vi "CSM - Running Log - DebugTool (CSMized).vi"() -> ()   [LabVIEW 2017]
doc: "Real-time tool for viewing the running log of the entire CSM program."
uses:
  Utility/_support/Periodic String Filter Level.ctl
  _Support/Typedef/_CSM_GlobalLog_MSG.ctl
  _Support/Typedef/_CSM_Response Source Message.ctl
  _Support/Typedef/_CSM_GlobalLog_MSG_TYPE.ctl
  _Support/GlobalEvent/GEvt-Generate with Rule Check.vi
  AdvanceAPI/CSM - Revert Arguments-Safe String.vi
  AdvanceAPI/CSM - Compact Multiple States.vi
  AdvanceAPI/CSM - Make String Arguments Safe.vi
  AdvanceAPI/CSM - Keywords.vi
  _Support/GlobalEvent/LogFilter/LogFilter - Check.vi
  _Support/GlobalEvent/FGV-GEvt Refs.vi
  _Shared/Trim Single-line Text.vi
  _Support/GlobalEvent/LogFilter/LogFilter.lvclass
  Communicable State Machine.lvlib
  addons/Logger/CSM File Logger.lvlib
  _Support/csm-tool-support.lvlib
  _csmHelper/API with lvcsm Support/CSM-Helper API with lvcsm Support.lvlib
panel:
  in  "Check Periodic Messages":bool
  in  "Filter Peroid Logs":bool
  in  "Record.Stop":bool
  in  "Record.Start":bool
  in  "BackTop":bool
  in  "Toolbar.History Length(char)":i32=50000 caption="History(char)" min=1000 max=100000000 step=1
  in  "Clear":bool
  in  "CSM":string(combo)
  in  "Search Button":bool
  in  "Toolbar.Open BD":bool
  in  "Toolbar.Open FP":bool
  in  "Periodic":bool
  in  "Check Peroid(s)":dbl=3.0
  in  "Threashold(#/s)":dbl=0.5
  in  "Periodic Info":bool=TRUE
  out "Handling Speed(#/s)":dbl
  in  "Level":T1
  out "LogInQ":i32
  out "State History":string
  in  "Tab":enum32{"Error History", "Broadcast Registry"}(tab)
  out "Error History":string
  out "Broadcast Registry":string[][](table)
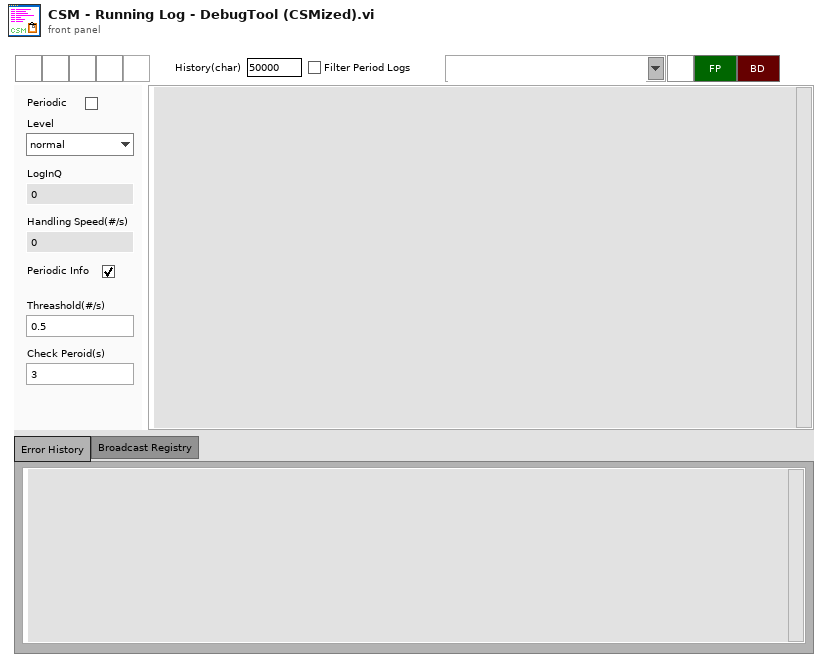
[diagram p1: front panel]
types:
  T1 = typedef "Communicable State Machine.lvlib/Periodic String Filter Level.ctl" = enum16{"normal", "L1", "L2", "L3", "L4"}
  T2 = enum32{"Invalid", "Standard", "Closed", "Hidden", "Minimized", "Maximized"}
  T3 = enum32{"invalid app kind", "Development System", "Run Time System", "Student Edition", "Embedded LabVIEW", "Evaluation", "Custom"}
  T4 = typedef "Communicable State Machine.lvlib/_CSM_Response Source Message.ctl" = cluster{"‘State":string, "’Arguments":string, "’Error":errorcluster}
  T5 = typedef "LVPoint32TypeDef.ctl" = cluster{"Horizontal":i32, "Vertical":i32}
  T6 = cluster{"Shift":bool, "Ctrl":bool, "Alt":bool, "Cmd":bool, "Opt":bool}
  T7 = cluster{"Core":cluster{"Current VI Reference":refnum<vi>, "Close Panel on Exit?":bool}, "Toolbar.Advance":refnum<vi>[], "LoggerWatchDogQueue":refnum<queue>, "LogFile":path}
  T8 = cluster{"Current VI Reference":refnum<vi>, "Close Panel on Exit?":bool}
  T9 = typedef "Communicable State Machine.lvlib/CSM - Broadcast Message Type.ctl" = enum16{"Status", "Interrupt(High)"}
  T10 = cluster{"Status":string, "Source CSM":string, "Target CSM":string, "Target API":string, "Priority":T9}[]
  T11 = cluster{"threashold(#/s)":dbl, "Check Peroid(s)":dbl}
  T12 = typedef "Communicable State Machine.lvlib/_CSM_GlobalLog_MSG.ctl" = cluster{"Name(\"\" to use uuid)":string, "Current State":string, "Arguments":string, "Source Message":T4, "Source Module":string, "Complete(T)/Start(F)":bool, "LogType":T13, "Time Stamp":timestamp}
  T13 = typedef "Communicable State Machine.lvlib/_CSM_GlobalLog_MSG_TYPE.ctl" = enum16{"User Log", "State Change", "Status", "Interrupt", "Register", "Unregister", "Error Log", "Module Created", "Module Destroyed"}
  T14 = cluster{"Threashold(#/s)":dbl, "Check Peroid(s)":dbl}
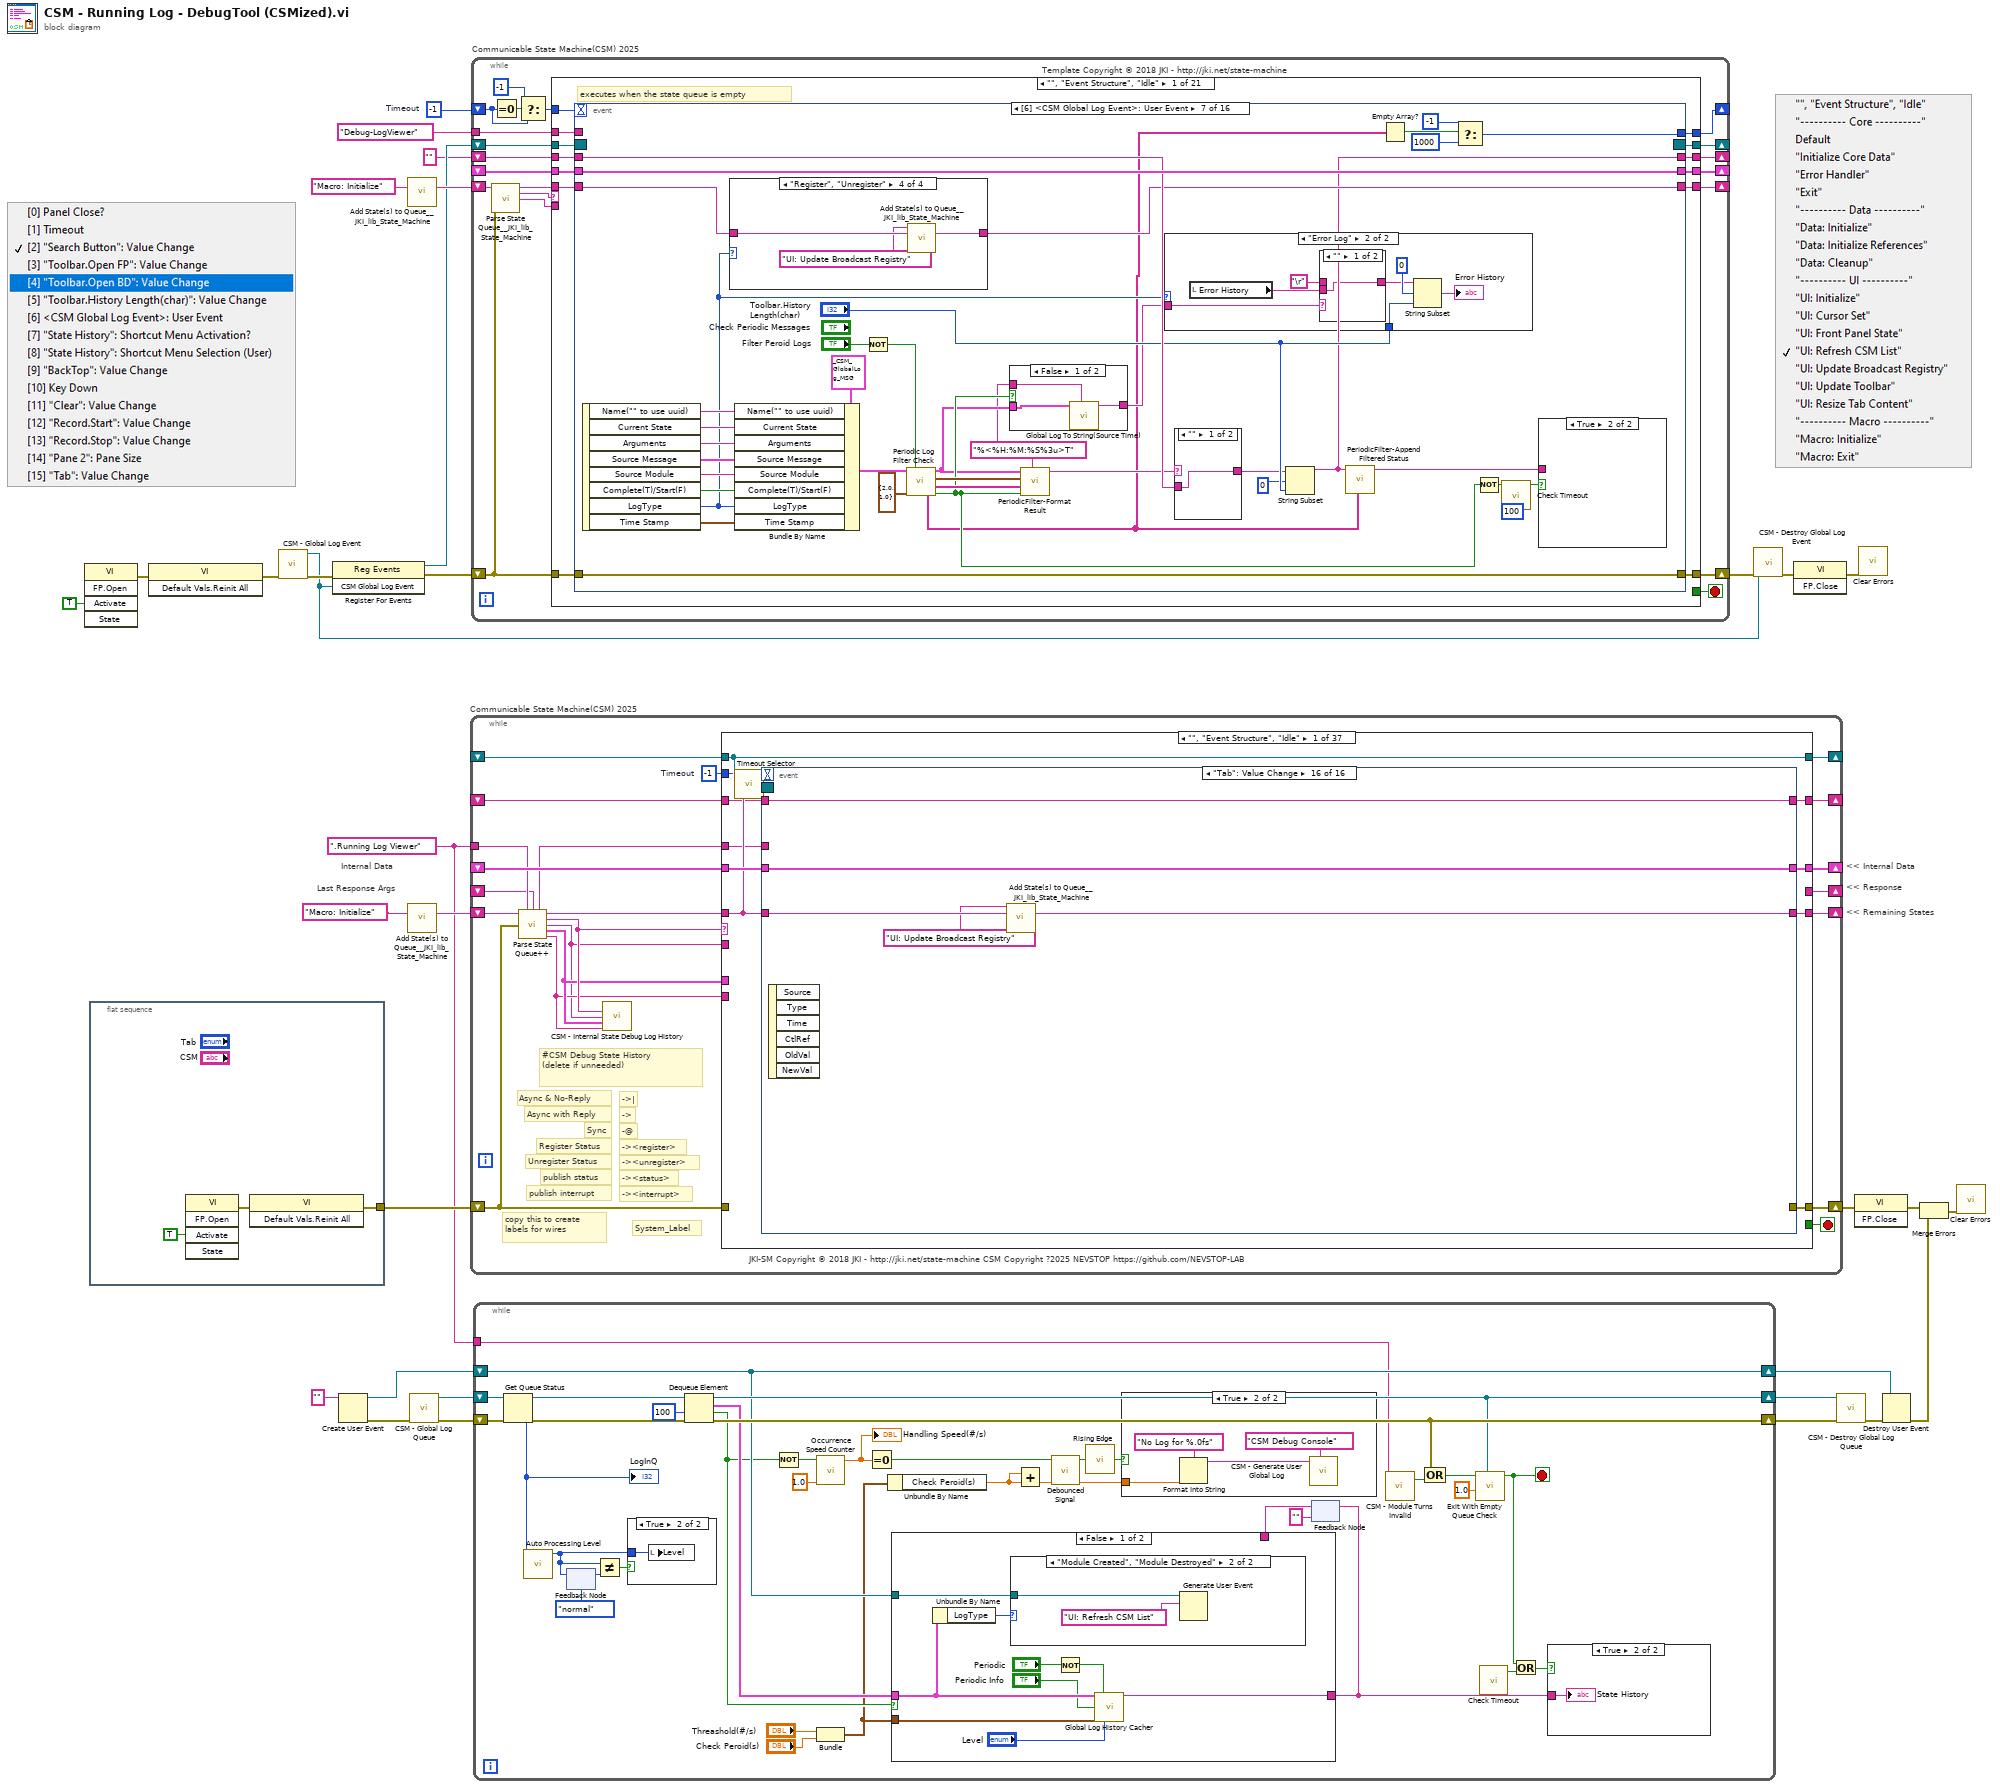
[diagram p0: block diagram]
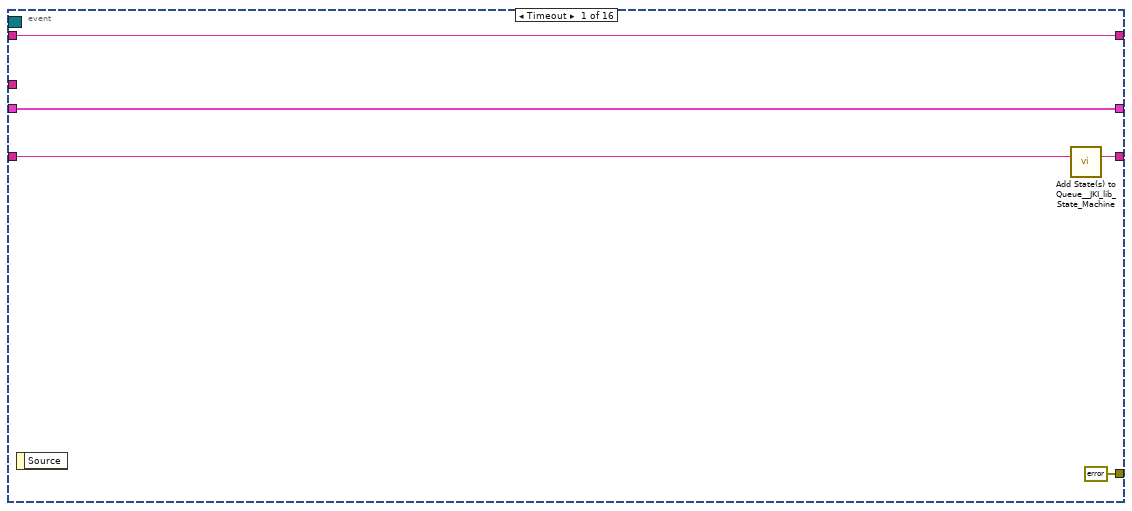
[diagram p7: hidden frame]
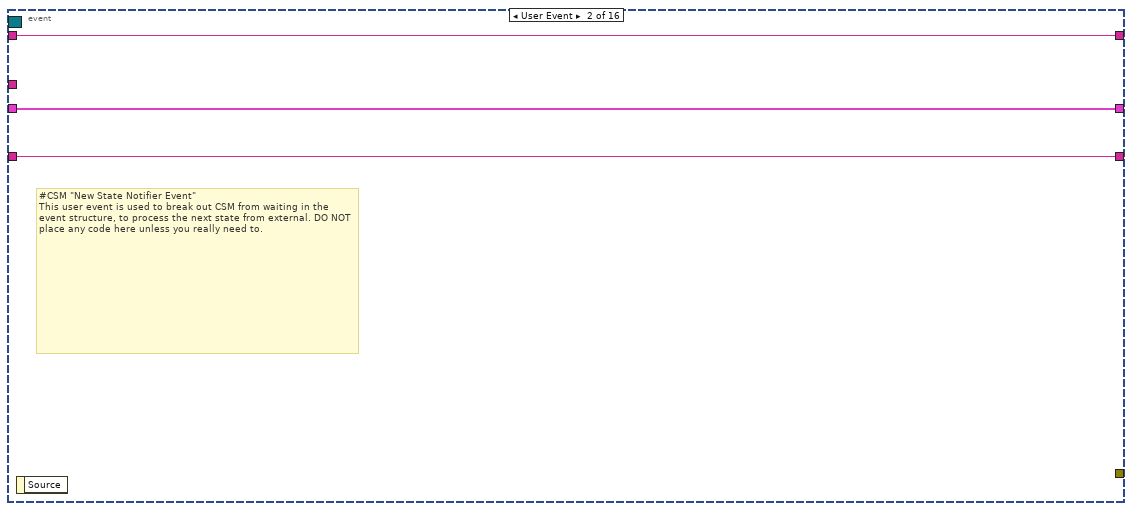
[diagram p8: hidden frame]
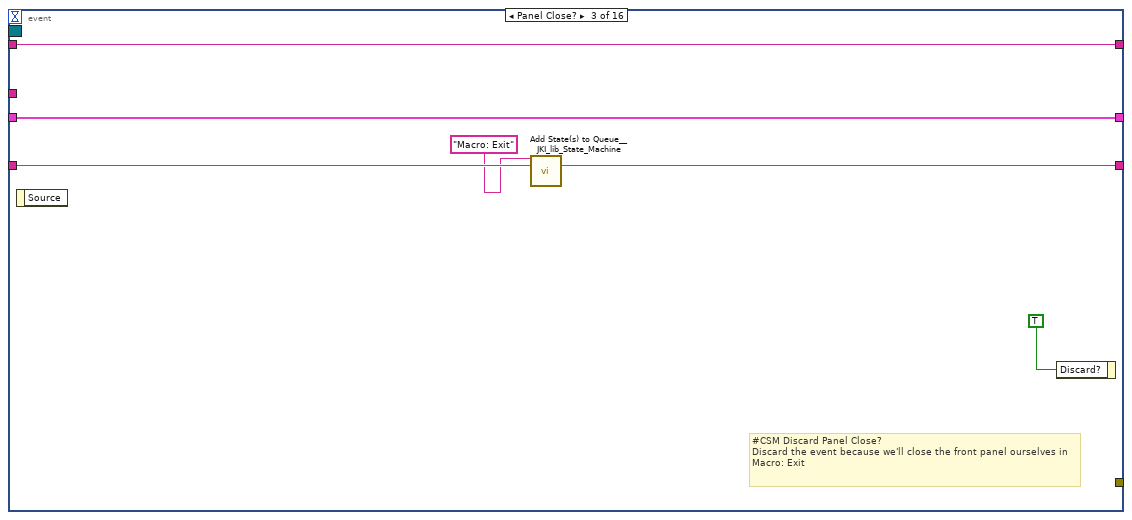
[diagram p9: hidden frame]
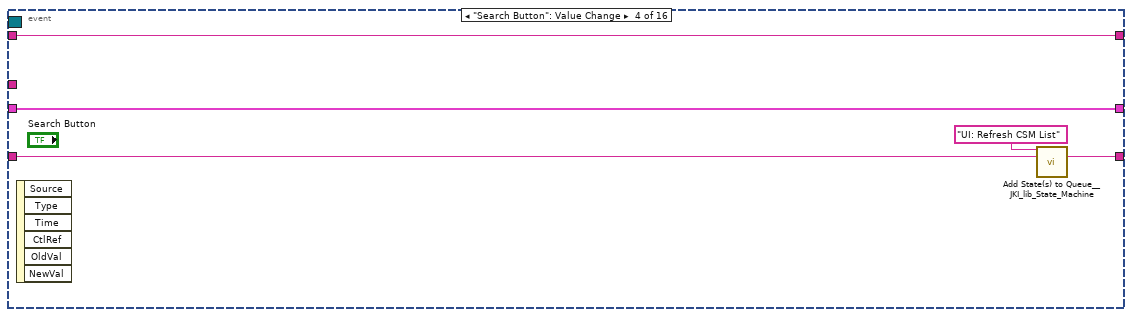
[diagram p10: hidden frame]
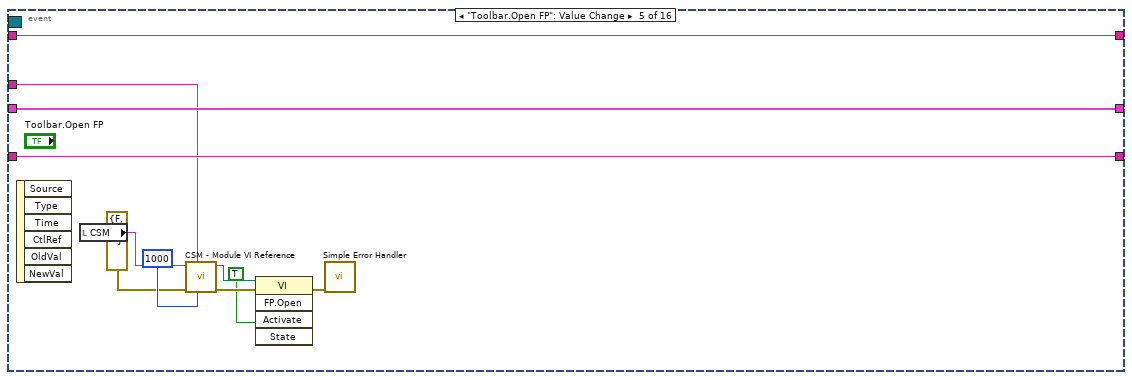
[diagram p11: hidden frame]
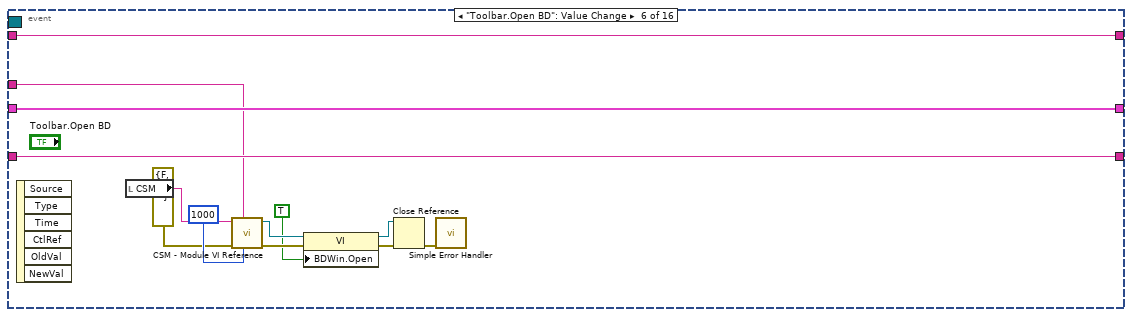
[diagram p12: hidden frame]
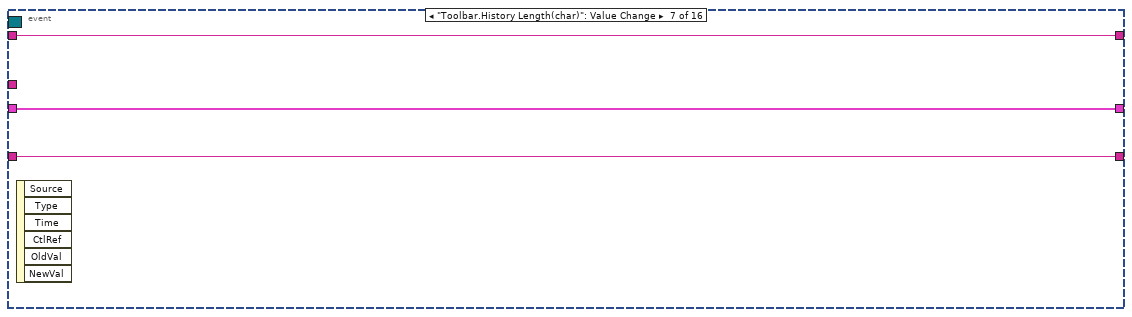
[diagram p13: hidden frame]
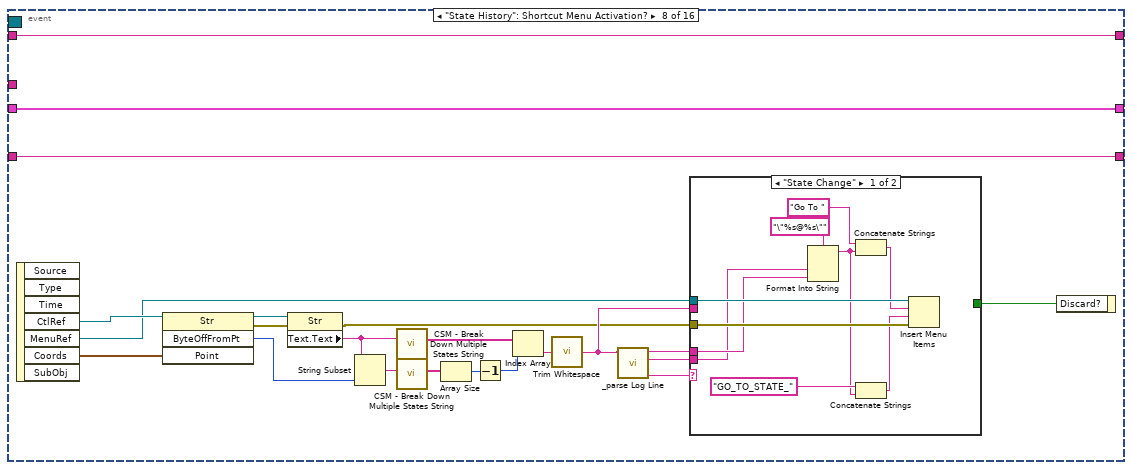
[diagram p14: hidden frame]
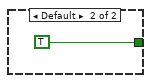
[diagram p15: hidden frame]
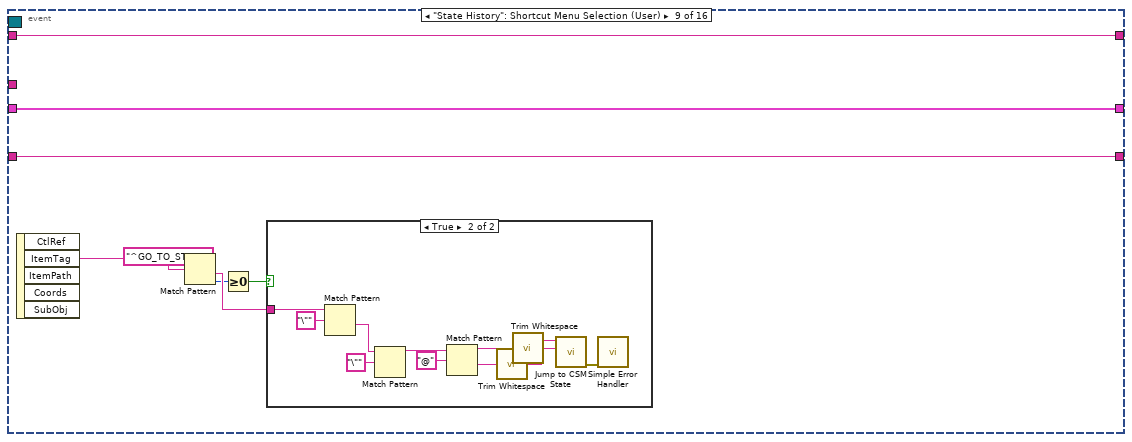
[diagram p16: hidden frame]
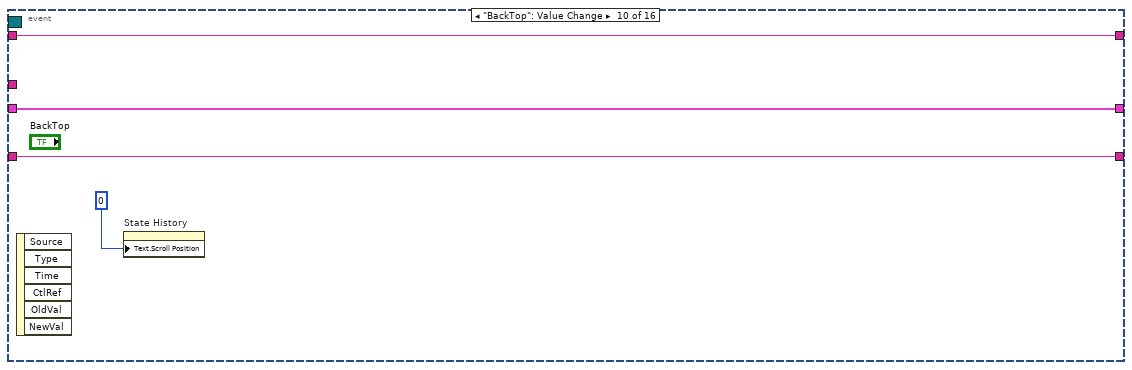
[diagram p18: hidden frame]
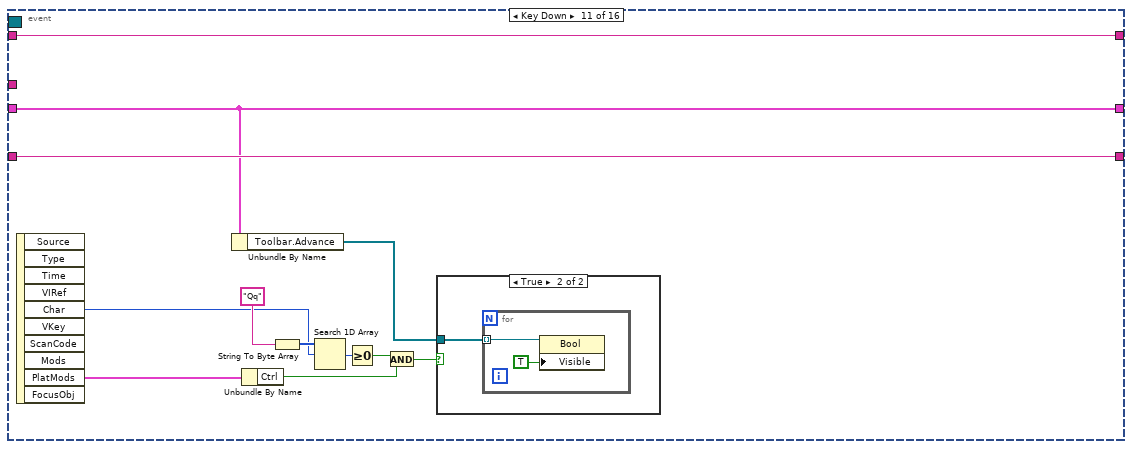
[diagram p19: hidden frame]
diagram:
  w7 = ".Running Log Viewer" ("Name(\"\" to use uuid)")
  w18 = -1  # Timeout
  # "Last Response Args"
  # "Internal Data"
  # "<< Internal Data"
  # "<< Response"
  # "<< Remaining States"
  n1 = invoke class="VI" method="FP.Open"("Activate"=TRUE ("Activate?")) -> (error out=w31:errorcluster)  [unwired: 4 in, 4 out]
  n2 = flat-sequence {
    tunnel: [w33] -> w15
    frame #0 {
      n3 = invoke class="VI" method="FP.Open"("Activate"=TRUE ("Activate?")) -> (error out=w35:errorcluster)  [unwired: 4 in, 4 out]
      n4 = invoke class="VI" method="Default Vals.Reinit All"(error in=w35) -> (error out=w33:errorcluster)  [unwired: 2 in, 2 out]
    }
  }
  n5 = invoke class="VI" method="Default Vals.Reinit All"(error in=w31) -> (error out=w25:errorcluster)  [unwired: 2 in, 2 out]
  n6 = call "CSM - Global Log Event.vi"("Error in"=w25) -> ("Error out"=w29:errorcluster, "CSM Global Log Event"=w28:refnum<user-event>)  [unwired: 9 in]
  n7 = register-events(error in=w29, w28) -> (reference out=w23:refnum<event-registration>, error out=w24:errorcluster)  [unwired: 1 in]
  n8 = Create User Event(user event datatype="" ("UserEvent")) -> (user event=w8:refnum<user-event>, error out=w9:errorcluster)  [unwired: 1 in]
  n9 = call <vilib>:"Add State(s) to Queue__JKI_lib_State_Machine.vi"("State(s) in (\"\")"="Macro: Initialize") -> ("States Out"=w27:string)  [unwired: 14 in]
  n10 = call <vilib>:"Add State(s) to Queue__JKI_lib_State_Machine.vi"("State(s) in (\"\")"="Macro: Initialize" ("Init State(\"Macro: Initialize\")")) -> ("States Out"=w17:string)  [unwired: 14 in]
  n11 = call "CSM - Global Log Queue.vi"("Error in"=w9) -> ("Error out"=w11:errorcluster, "GlobalEvent Queue"=w12:refnum<queue>)  [unwired: 9 in]
  n12 = while "Communicable State Machine(CSM) 2025" {
    shift-right: [w51] -> _
    shift-left: _ -> [w50]
    shift-right: [w54] -> w13
    shift-left: w15 -> [w48]
    shift-right: [w53] -> _
    shift-left: w17 -> [w55]
    tunnel: w7 -> [w44]
    shift-right: [w47] -> _
    shift-left: _ -> [w39]
    shift-right: [w46] -> _
    shift-left: _ -> [w45]
    shift-right: [w37] -> _
    shift-left: _ -> [w36]
    stop <- w52 stop-if-true
    w49 = -1  # Timeout
    # "#CSM Debug State History\n(delete if unneeded)"
    # "-><interrupt>"
    # "-><status>"
    # "-><unregister>"
    # "-><register>"
    # "-@"
    # "->"
    # "->|"
    # "publish interrupt"
    # "publish status"
    # "Unregister Status"
    # "Register Status"
    # "Sync"
    # "Async with Reply"
    # "Async & No-Reply"
    # "copy this to create labels for wires"
    # "System_Label"
    # "JKI-SM Copyright © 2018 JKI - http://jki.net/state-machine CSM Copyright ?2025 NEVSTOP https://github.com/NEVSTOP-LAB"
    n13 = call "Parse State Queue++.vi"("State Queue"=w55, "Name(\"\" to use uuid)"=w44, "Response Arguments"=w39, "Previous Error"=w48) -> ("Name Used"=w40:string, "Remaining States"=w56:string, "Current State"=w43:string, "Arguments"=w38:string, ">> Response Source Message >>"=w42:T4, ">> Source CSM >>"=w41:string)  [unwired: 6 in]
    n14 = call "CSM - Internal State Debug Log History.vi"("State"=w43, "Arguments (\"\")"=w38, ">> Response Source Message >>"=w42, "Source (\"\")"=w41) -> ()  [unwired: 11 in, 1 out]
    n15 = case shown="\"\", \"Event Structure\", \"Idle\"" w43 {
      selector: w43 -> [_ _ _ w237 _ _ _ _ _ _ _ _ _ _ _ _ _ _ _ _ _ _ _ _ _ _ _ _ _ _ _ _ _ _ _ _ _]
      tunnel: w56 -> [w60 w227 w233 w243 w250 w257 w284 w293 w301 w312 w322 w336 w342 w347 w356 w364 w372 w377 w385 w390 w395 w400 w407 w419 w490 w498 w525 w548 w554 w560 w572 w576 w581 w585 w590 w595 w600]
      tunnel: w38 -> [_ _ _ _ _ w255 w280 w288 w297 w306 _ _ _ _ _ _ _ _ _ _ _ _ w403 w414 _ _ _ _ _ _ _ _ _ _ _ _ _]
      tunnel: w50 -> [w66 w226 w230 w241 w249 w263 w285 w291 w299 w310 w321 w330 w340 w345 _ w360 w368 w375 w384 w389 w393 w398 w405 w416 w489 w497 w508 w547 w552 w558 w570 w575 w580 w584 w588 w593 w598]
      tunnel: [w65 _ w231 w235 w251 errorcluster {"status"=FALSE, "code"=0, "source"=""} ("error out") w277 w287 w295 w309 _ _ _ _ _ w365 w369 _ w379 w388 _ _ w404 w417 w491 w493 w526 w549 _ _ _ _ _ _ _ _ _] -> w54
      tunnel: w48 -> [_ _ w231 w236 w251 w261 w278 w289 w296 _ _ _ _ _ _ w365 _ _ _ _ _ _ _ _ w491 _ w526 w549 _ _ _ _ _ _ _ _ _]
      tunnel: [w67 w227 w232 w242 w250 w259 w283 w292 w300 w313 w322 w335 w341 w346 w355 w364 w371 w376 w385 w390 w394 w399 w406 w418 w490 w498 w525 w548 w553 w559 w571 w576 w581 w585 w589 w594 w599] -> w53
      tunnel: [_ _ _ _ _ _ TRUE _ _ _ _ _ TRUE _ _ _ _ _ _ _ _ _ _ _ _ _ _ _ _ _ _ _ _ _ _ _ _] -> w52
      tunnel: [w64 w226 w230 w241 w249 w263 w285 w291 w299 w311 w321 w334 w340 w345 w354 w358 w368 w375 w384 w389 w393 w398 w405 w416 w489 w497 w508 w547 w552 w558 w570 w575 w580 w584 w588 w593 w598] -> w51
      tunnel: w49 -> [w62 _ _ _ _ _ _ _ _ _ _ _ _ _ _ _ _ _ _ _ _ _ _ _ _ _ _ _ _ _ _ _ _ _ _ _ _]
      tunnel: w41 -> [_ _ _ _ _ w254 _ _ _ w307 _ _ _ _ _ _ _ _ _ _ _ _ _ _ _ _ _ _ _ _ _ _ _ _ _ _ _]
      tunnel: w42 -> [_ _ _ _ _ w253 _ _ _ w308 _ _ _ _ _ _ _ _ _ _ _ _ _ _ _ _ _ _ _ _ _ _ _ _ _ _ _]
      tunnel: [_ _ _ "" w245 _ _ _ _ _ _ _ _ _ _ _ _ _ _ _ _ _ _ _ _ _ _ _ _ _ _ _ "API1 Response" _ _ _ _] -> w47
      tunnel: [w63 w225 w229 w239 w248 w262 w281 w290 w298 w314 w320 w324 w338 w344 w352 w363 w367 w374 w383 w387 w392 w397 w402 w413 w488 w496 w524 w546 w551 w556 w563 w574 w579 w583 w587 w592 w597] -> w46
      tunnel: w45 -> [w63 w225 w229 w239 w248 w262 w281 w290 w298 w314 w320 w324 w338 w344 w352 w363 w367 w374 _ w387 w392 w397 w402 w413 w488 w496 w524 w546 w551 w556 w563 w574 w579 w583 w587 w592 w597]
      tunnel: w40 -> [w59 _ _ w238 _ _ w279 _ _ _ _ _ _ _ _ _ _ _ w382 _ _ _ _ _ _ _ _ _ _ _ _ _ _ _ _ _ _]
      tunnel: [w58 w224 w228 w234 w244 w252 w276 w286 w294 w302 w319 w323 w337 w343 w348 w357 w366 w373 w378 w386 w391 w396 w401 w412 w480 w492 w507 w533 w550 w555 w561 w573 w577 w582 w586 w591 w596] -> w37
      tunnel: w36 -> [w57 w224 w228 w234 w244 w252 w276 w286 w294 w302 w319 w323 w337 w343 w348 w357 w366 w373 w378 w386 w391 w396 w401 w412 w480 w492 w507 w533 w550 w555 w561 w573 w577 w582 w586 w591 w596]
      frame "", "Event Structure", "Idle" {
        n16 = call "Timeout Selector.vi"("Remaining States"=w60, "Timeout Expected"=w62) -> ("Timeout"=w61:i32)  [unwired: 5 in]
        n17 = event shown="[15] \"Tab\": Value Change" {
          selector: w63 -> [_ _ _ _ _ _ _ _ _ _ _ _ _ _ _ _]
          dyn-events: _ -> [_ _ _ _ _ _ _ _ _ _ _ _ _ _ _ _]
          timeout: w61 -> [_ _ _ _ _ _ _ _ _ _ _ _ _ _ _ _]
          tunnel: w60 -> [w72 w74 w81 w85 w97 w110 w113 w135 w154 w169 w181 w187 w191 w206 w214 w220]
          tunnel: [w71 w74 w80 w84 w97 w110 w113 w135 w154 w169 w181 w187 w190 w205 w215 w221] -> w67
          tunnel: w66 -> [w70 w75 w79 w86 w96 w109 w112 w134 w153 w168 w171 w186 w193 w208 w218 w223]
          tunnel: [errorcluster {"status"=FALSE, "code"=0, "source"=""} ("error out") _ _ _ _ _ _ _ _ _ _ _ w188 _ _ _] -> w65
          tunnel: [w70 w75 w79 w86 w96 w109 w112 w134 w153 w168 w171 w186 w192 w207 w218 w223] -> w64
          tunnel: w59 -> [_ _ _ _ w88 w99 _ _ _ _ _ _ _ _ _ _]
          tunnel: [w68 w73 w76 w82 w87 w98 w111 w114 w147 w166 w170 w185 w203 w213 w217 w222] -> w58
          tunnel: w57 -> [w68 w73 w76 w82 w87 w98 w111 w114 w147 w166 w170 _ w203 w213 w217 w222]
          event Timeout {
            n18 = event-data() -> ()  [unwired: 1 in, 1 out]
            n19 = call <vilib>:"Add State(s) to Queue__JKI_lib_State_Machine.vi"("State(s) in (\"\")"=w72) -> ("States Out"=w71:string)  [unwired: 14 in]
          }
          event User Event {
            # "#CSM \"New State Notifier Event\"\nThis user event is used to break out CSM from waiting in the event structure, to process the next state from external. DO NOT place any code here unless you really need to."
            n20 = event-data() -> ()  [unwired: 1 in, 1 out]
          }
          event Panel Close? {
            # "#CSM Discard Panel Close?\nDiscard the event because we'll close the front panel ourselves in Macro: Exit"
            n21 = event-data() -> ()  [unwired: 1 in, 1 out]
            n22 = call <vilib>:"Add State(s) to Queue__JKI_lib_State_Machine.vi"("State(s) in Front (\"\")"="Macro: Exit", "State(s) in (\"\")"=w81) -> ("States Out"=w80:string)  [unwired: 13 in]
            n23 = event-data("Discard?"=TRUE) -> ()  [unwired: 1 in, 1 out]
          }
          event "Search Button": Value Change {
            n24 = event-data() -> ()  [unwired: 1 in, 6 out]
            n25 = call <vilib>:"Add State(s) to Queue__JKI_lib_State_Machine.vi"("State(s) in Front (\"\")"="UI: Refresh CSM List" ("State(s) in Front (\"\")"), "State(s) in (\"\")"=w85) -> ("States Out"=w84:string)  [unwired: 13 in]
          }
          event "Toolbar.Open FP": Value Change {
            n26 = event-data() -> ()  [unwired: 1 in, 6 out]
            n27 = local read "CSM"() -> (w93:string)
            n28 = call "CSM - Module VI Reference.vi"("Response Timeout(-2 using Global Settings)"=1000 ("Response Timeout(5000ms)"), "Current Module(\"\" to generate a ID)"=w88, "error in (no error)"=errorcluster {"status"=FALSE, "code"=0, "source"=""}, "CSM Name"=w93) -> ("error out"=w95:errorcluster, "CSM Module VIRef"=w94:refnum<vi>)  [unwired: 6 in]
            n29 = invoke on="Invoke Node" class="VI" method="FP.Open"(reference=w94, error in=w95, "Activate"=TRUE ("Activate?")) -> (error out=w92:errorcluster)  [unwired: 2 in, 4 out]
            n30 = call <vilib>:"Simple Error Handler.vi"("error in (no error)"=w92) -> ()  [unwired: 4 in, 5 out]
          }
          event "Toolbar.Open BD": Value Change {
            n31 = event-data() -> ()  [unwired: 1 in, 6 out]
            n32 = local read "CSM"() -> (w104:string)
            n33 = call "CSM - Module VI Reference.vi"("Response Timeout(-2 using Global Settings)"=1000 ("Response Timeout(5000ms)"), "Current Module(\"\" to generate a ID)"=w99, "error in (no error)"=errorcluster {"status"=FALSE, "code"=0, "source"=""}, "CSM Name"=w104) -> ("error out"=w108:errorcluster, "CSM Module VIRef"=w105:refnum<vi>)  [unwired: 6 in]
            n34 = property class="VI"(reference=w105, error in=w108, "BDWin.Open"=TRUE ("Block Diagram Window:Open")) -> (reference out=w106:refnum<vi>, error out=w107:errorcluster)
            n35 = Close Reference(reference=w106, error in (no error)=w107) -> (error out=w103:errorcluster)
            n36 = call <vilib>:"Simple Error Handler.vi"("error in (no error)"=w103) -> ()  [unwired: 4 in, 5 out]
          }
          event "Toolbar.History Length(char)": Value Change {
            n37 = event-data() -> ()  [unwired: 1 in, 6 out]
          }
          event "State History": Shortcut Menu Activation? {
            n38 = event-data() -> ("CtlRef"=w118:refnum<vi>, "MenuRef"=w116:refnum<k9>, "Coords"=w117:T5)  [unwired: 1 in, 4 out]
            n39 = invoke class="Str" method="ByteOffFromPt"(reference=w118, "Point"=w117) -> (reference out=w119:refnum<vi>, error out=w121:errorcluster, "ByteOffFromPt"=w120:i32)  [unwired: 2 in, 1 out]
            n40 = property class="Str"(reference=w119, error in=w121) -> (error out=w129:errorcluster, "Text.Text"=w123:string)  [unwired: 1 out]
            n41 = String Subset(string=w123, length (rest)=w120) -> (substring=w122:string)  [unwired: 1 in]
            n42 = call "CSM - Break Down Multiple States String.vi"("States"=w123) -> ("Multiple States"=w124:string[])  [unwired: 10 in]
            n43 = call "CSM - Break Down Multiple States String.vi"("States"=w122) -> ("Multiple States"=w125:string[])  [unwired: 10 in]
            n44 = Array Size(array=w125) -> (size(s)=w126:i32)
            n45 = Decrement(x=w126) -> (x-1=w127:i32)
            n46 = Index Array(array=w124, index=w127) -> (element=w128:string)
            n47 = call <vilib>:"Trim Whitespace.vi"("string"=w128) -> ("trimmed string"=w130:string)  [unwired: 1 in]
            n48 = call "_parse Log Line.vi"("string"=w130) -> ("LogType"=w131:string, "State"=w133:string, "CSM"=w132:string)  [unwired: 8 in]
            n49 = case shown="\"State Change\"" w131 {
              tunnel: w116 -> [w145 _]
              tunnel: w130 -> [_ _]
              tunnel: w129 -> [w143 _]
              tunnel: [_ TRUE] -> w115
              tunnel: w132 -> [w141 _]
              tunnel: w133 -> [w140 _]
              frame "State Change" {
                n50 = Format Into String(format string="\"%s@%s\"", w140, w141) -> (resulting string=w136:string)  [unwired: 2 in, 1 out]
                n51 = Concatenate Strings("Go To " ("format string"), w136) -> (w139:string)
                n52 = Concatenate Strings("GO_TO_STATE_" ("item tags"), w136) -> (w137:string)
                n53 = Insert Menu Items(6:w143, 7:w137, 8:w139, 9:w145) -> ()  [unwired: 2 in, 3 out]
              }
              frame Default {
              }
            }
            n54 = event-data("Discard?"=w115) -> ()  [unwired: 1 in, 1 out]
          }
          event "State History": Shortcut Menu Selection (User) {
            n55 = event-data() -> ("ItemTag"=w148:string)  [unwired: 1 in, 4 out]
            n56 = Match Pattern(string=w148, regular expression="^GO_TO_STATE") -> (after substring=w152:string, offset past match=w150:i32)  [unwired: 1 in, 2 out]
            n57 = Greater Or Equal To 0?(x=w150) -> (x >= 0?=w151:bool)
            n58 = case shown="True" w151 {
              tunnel: w152 -> [_ w165]
              frame False {
              }
              frame True {
                n59 = Match Pattern(string=w165, regular expression="\"") -> (after substring=w162:string)  [unwired: 1 in, 3 out]
                n60 = Match Pattern(string=w162, regular expression="\"") -> (before substring=w161:string)  [unwired: 1 in, 3 out]
                n61 = Match Pattern(string=w161, regular expression="@") -> (before substring=w159:string, after substring=w158:string)  [unwired: 1 in, 2 out]
                n62 = call <vilib>:"Trim Whitespace.vi"("string"=w158) -> ("trimmed string"=w156:string)  [unwired: 1 in]
                n63 = call <vilib>:"Trim Whitespace.vi"("string"=w159) -> ("trimmed string"=w157:string)  [unwired: 1 in]
                n64 = call "Jump to CSM State.vi"("State"=w157, "Name"=w156) -> ("Error out"=w155:errorcluster)  [unwired: 9 in]
                n65 = call <vilib>:"Simple Error Handler.vi"("error in (no error)"=w155) -> ()  [unwired: 4 in, 5 out]
              }
            }
          }
          event "BackTop": Value Change {
            n66 = event-data() -> ()  [unwired: 1 in, 6 out]
            n67 = property on="State History" class="Str"("Text.Scroll Position"=u32 0) -> ()  [unwired: 2 in, 2 out]
          }
          event Key Down {
            n68 = event-data() -> ("Char"=w173:i16, "PlatMods"=w172:T6)  [unwired: 1 in, 8 out]
            n69 = Unbundle By Name(w171) -> ("Toolbar.Advance"=w180:refnum<vi>[])
            n70 = Unbundle By Name(w172) -> ("Ctrl"=w178:bool)
            n71 = String To Byte Array(string="Qq") -> (unsigned byte array=w176:u8[])
            n72 = Search 1D Array(1D array=w176, element=w173) -> (index of element=w175:i32)  [unwired: 1 in]
            n73 = Greater Or Equal To 0?(x=w175) -> (x >= 0?=w174:bool)
            n74 = And(x=w174, y=w178) -> (x .and. y?=w179:bool)
            n75 = case shown="True" w179 {
              tunnel: w180 -> [_ w182]
              frame False {
              }
              frame True {
                n76 = for {
                  tunnel: w182 -> [w184] mode=indexing
                  n77 = property class="Bool"(reference=w184, "Visible"=TRUE) -> ()  [unwired: 1 in, 2 out]
                }
              }
            }
          }
          event "Clear": Value Change {
            w185 = "" ("String Cache")
            n78 = event-data() -> ()  [unwired: 1 in, 6 out]
            n79 = local write "State History"(w185) -> ()
            n80 = local write "Error History"(w185) -> ()
          }
          event "Record.Start": Value Change {
            n81 = event-data() -> ()  [unwired: 1 in, 6 out]
            n82 = Unbundle By Name(w193) -> ("Core.Current VI Reference"=w196:refnum<vi>)
            n83 = property class="VI"(reference=w196) -> (error out=w197:errorcluster, "OwningApp"=w198:refnum<vi>)  [unwired: 1 in, 1 out]
            n84 = property class="App"(reference=w198, error in=w197) -> (error out=w200:errorcluster, "Project.ActiveProject"=w199:refnum<vi>)  [unwired: 1 out]
            n85 = property class="Project"(reference=w199, error in=w200) -> ("Name"=w201:string)  [unwired: 2 out]
            n86 = String To Path(string=w201) -> (path=w202:path)
            n87 = call "CSM - Start File Logger.vi"("Log File Path"=w202) -> ("Error out"=w188:errorcluster, "LogFile"=w195:path, "WatchDogQueue"=w194:refnum<queue>)  [unwired: 8 in]
            n88 = Bundle By Name(cluster=w193, "LoggerWatchDogQueue"=w194, "LogFile"=w195) -> (w192:T7)
            n89 = call <vilib>:"Add State(s) to Queue__JKI_lib_State_Machine.vi"("State(s) in Front (\"\")"="UI: Update Toolbar" ("State(s) in Front (\"\")"), "State(s) in (\"\")"=w191) -> ("States Out"=w190:string)  [unwired: 13 in]
          }
          event "Record.Stop": Value Change {
            n90 = event-data() -> ()  [unwired: 1 in, 6 out]
            n91 = Unbundle By Name(w208) -> ("LoggerWatchDogQueue"=w212:refnum<queue>)
            n92 = Release Queue(queue=w212, force destroy? (F)=TRUE) -> (error out=w210:errorcluster)  [unwired: 1 in, 2 out]
            n93 = call <vilib>:"Clear Errors.vi"("error in (no error)"=w210) -> ()  [unwired: 5 in, 2 out]
            n94 = Bundle By Name(cluster=w208, "LogFile"=path "") -> (w207:T7)
            n95 = call <vilib>:"Add State(s) to Queue__JKI_lib_State_Machine.vi"("State(s) in Front (\"\")"="UI: Update Toolbar" ("State(s) in Front (\"\")"), "State(s) in (\"\")"=w206) -> ("States Out"=w205:string)  [unwired: 13 in]
          }
          event Pane Size {
            n96 = event-data() -> ()  [unwired: 1 in, 6 out]
            n97 = call <vilib>:"Add State(s) to Queue__JKI_lib_State_Machine.vi"("State(s) in (\"\")"=w214, "State(s) at Back (\"\")"="UI: Resize Tab Content" ("State(s) in Front (\"\")")) -> ("States Out"=w215:string)  [unwired: 13 in]
          }
          event "Tab": Value Change {
            n98 = event-data() -> ()  [unwired: 1 in, 6 out]
            n99 = call <vilib>:"Add State(s) to Queue__JKI_lib_State_Machine.vi"("State(s) in Front (\"\")"="UI: Update Broadcast Registry" ("State(s) in Front (\"\")"), "State(s) in (\"\")"=w220) -> ("States Out"=w221:string)  [unwired: 13 in]
          }
        }
      }
      frame "CSM Documentation" {
        # "#CSM State Syntax\n\n// Comment line, all text to the right of “//” will be ignored\n// Local Message Example\nDoSth: DoA >> Arguments\n\n// Sync Call Example\nAPI: xxxx >> Arguments -@ TargetModule\n\n// Async Call Example\nAPI: xxxx >> Arguments -> TargetModule\n\n// Async Call without Reply Example\nAPI: xxxx >> Arguments ->| TargetModule\n\n// Broadcast normal status:\nStatus >> StatusArguments  -><status>\n\n// Broadcast Interrupt status:\nInterrupt >> StatusArguments  -><interrupt>\n\n// Register Source Module's status to Handler Module\nStatus@Source Module >> Handler Module@Handler Module -><register>\n\n// Unegister Source Module's status\nStatus@Source Module >> Handler Module -><unregister>"
        # "#CSM README FIRST\n\nCommunicable State Machine(CSM) is a LabVIEW application framework that builds upon JKI State Machine(JKISM). It follows the pattern of JKISM and extends the keywords to describe message communication between modules, including concepts such as Sync-Message, Async-Message, Subscription/Unsubscription of status - essential elements for creating reusable code modules. For more information, please visit the CSM wiki: https://nevstop-lab.github.io/CSM-Wiki/\n\nFor instructions on JKI State Machine, visit: \n    http://jki.net/state-machine/\nFor information about CSM, visit: \n    https://github.com/NEVSTOP-LAB"
        # "#CSM \"Documentation\"\nCase for holding CSM Documenation"
      }
      frame "---------- Core ----------" {
        # "#CSM \"Category Seperator\"\nDo not put any code in this frame."
        n100 = call <vilib>:"Add State(s) to Queue__JKI_lib_State_Machine.vi"("State(s) in (\"\")"=w233) -> ("States Out"=w232:string)  [unwired: 14 in]
      }
      frame Default {
        # "#CSM \"Default\"\nthis is used to capture unhandled states and typos"
        n101 = call "CSM Unhandled State Error.vi"("error in (no error)"=w236, "Current State"=w237, "CSM Name"=w238) -> ("error out"=w235:errorcluster)  [unwired: 8 in]
        n102 = call <vilib>:"Add State(s) to Queue__JKI_lib_State_Machine.vi"("State(s) in (\"\")"=w243) -> ("States Out"=w242:string)  [unwired: 14 in]
      }
      frame "VI Reference" {
        n103 = Unbundle By Name(w249) -> ("Core"=w247:T8)
        n104 = Unbundle By Name(w247) -> ("Current VI Reference"=w246:refnum<vi>)
        n105 = call "CSM - Convert Data to HexStr.vi"("Variant"=w246) -> ("HEX String (0-9,A-F)"=w245:string)  [unwired: 8 in]
      }
      frame "Error Handler" {
        # "#CSM Disable this error dialog if you need"
        # "#CSM \"Error Handler\"\nYou can also output any states to clean-up after errors occur"
        # "Clear error"
        n106 = case shown="Error" w261 {
          selector: w261 -> [_ w270]
          tunnel: [w268 w272] -> w258
          tunnel: w257 -> [w268 w271]
          tunnel: [w267 w270] -> w256
          tunnel: w255 -> [w269 _]
          tunnel: w254 -> [_ _]
          tunnel: w253 -> [_ _]
          frame No Error {
            n107 = call "CSM - Convert Argument to Error.vi"("Argument"=w269) -> ("error"=w267:errorcluster)  [unwired: 4 in]
            n108 = flat-sequence {
              frame #0 {
                # "#CSM External Error Handler Case\nUsually, it's because This CSM register others' \"Error Occurred\" status with \"Error Handler\". If other CSM have any error, the error will be passed here for central handling."
              }
            }
          }
          frame Error {
            # "#CSM Internal Error Handler Case \nIf any error Occurred, \"Error Occurred\" \nstatus update will be broadcasted to system.\nParameter is Error Cluster."
            n109 = call "CSM - Convert Error to Argument.vi"("error"=w270) -> ("Argument"=w274:string)  [unwired: 4 in]
            n110 = call <vilib>:"Build State String with Arguments__JKI_lib_State_Machine.vi"("Arguments (\"\")"=w274, "State"="Error Occurred" ("Status with Arguments")) -> ("State with Arguments"=w273:string)  [unwired: 4 in]
            n111 = call "CSM - Broadcast Status Change.vi"("Status with Arguments"=w273, "State Queue"=w271) -> ("Remaining States"=w272:string)  [unwired: 13 in]
          }
        }
        n112 = disable-structure shown="Enabled" {
          disable-tunnel: w256 -> [w265 w266]
          frame Enabled {
            # "Unhandled Error -- Display it"
            n113 = call <vilib>:"General Error Handler.vi"("error in (no error)"=w265) -> ()  [unwired: 10 in, 5 out]
          }
          frame Disabled {
            n114 = call <vilib>:"Clear Errors.vi"("error in (no error)"=w266) -> ()  [unwired: 5 in, 2 out]
          }
        }
        n115 = call <vilib>:"Add State(s) to Queue__JKI_lib_State_Machine.vi"("State(s) in Front (\"\")"="// Post Error States", "State(s) in (\"\")"=w258) -> ("States Out"=w259:string)  [unwired: 13 in]
      }
      frame "Critical Error" {
        # "#CSM \"Critical Error\"\nWhen any un-recoverable error occurs, CSM goes into this case."
        # "#CSM Stop in Critical Error\nWhen Critical Error occurs, Stop the loop immediately. Do NOT change this unless you fully understand the impact."
        n116 = call "CSM Critical Error.vi"("error in (no error)"=w278, "Arugments(as Reason)"=w280, "CSM Name"=w279) -> ("error out"=w277:errorcluster)  [unwired: 8 in]
        n117 = call <vilib>:"Add State(s) to Queue__JKI_lib_State_Machine.vi"("State(s) in (\"\")"=w284) -> ("States Out"=w283:string)  [unwired: 14 in]
      }
      frame "Target Timeout Error" {
        # "#CSM \"Target Timeout Error\"\nWhen This CSM could not get the sync-call response in time, This CSM goes into this case."
        n118 = call "CSM Target Timeout Error.vi"("error in (no error)"=w289, "Arguments(as CSM Name)"=w288) -> ("error out"=w287:errorcluster)  [unwired: 9 in]
        n119 = call <vilib>:"Add State(s) to Queue__JKI_lib_State_Machine.vi"("State(s) in (\"\")"=w293) -> ("States Out"=w292:string)  [unwired: 14 in]
      }
      frame "Target Error" {
        # "#CSM \"Target Error\"\nWhen This CSM try to communicate with an un-existed CSM, This CSM goes into this case."
        n120 = call "CSM Target Error.vi"("error in (no error)"=w296, "Arguments(as CSM Name)"=w297) -> ("error out"=w295:errorcluster)  [unwired: 9 in]
        n121 = call <vilib>:"Add State(s) to Queue__JKI_lib_State_Machine.vi"("State(s) in (\"\")"=w301) -> ("States Out"=w300:string)  [unwired: 14 in]
      }
      frame "Async Response", "Response" {
        # "#CSM \"Async Response\"\nHandle Async-call Response (\"Async Response\" for ->)"
        # "#CSM \"Response\"\nHandle Sync-call Response (\"Response\" for -@)"
        n122 = Unbundle(w308) -> ("‘State"=w305:string, "’Arguments"=w304:string, "’Error"=w303:errorcluster)
        n123 = case shown="Default" w305 {
          tunnel: [w315] -> w313
          tunnel: w312 -> [w316]
          tunnel: [w318] -> w311
          tunnel: w310 -> [w318]
          tunnel: [w317] -> w309
          tunnel: w303 -> [w317]
          tunnel: w307 -> [_]
          tunnel: w306 -> [_]
          tunnel: w304 -> [_]
          frame Default {
            # "#CSM Response Comments\nAfter Message is executed, CSM goes to this state for receive the response.\n    For Async Message(->), \"Async Response\" is used. This CSM will goes to \"Async Message Posted\" immediately and receive the \"Async Response\" after the callee finishes the message.\n    For Sync Message(@),  This CSM will wait until the message is done and immediately goes to \"Response\""
            n124 = call <vilib>:"Add State(s) to Queue__JKI_lib_State_Machine.vi"("State(s) in (\"\")"=w316) -> ("States Out"=w315:string)  [unwired: 14 in]
          }
        }
      }
      frame "Async Message Posted" {
        # "#CSM \"Async Message Posted\"\nAfter Async Message is posted (-> or ->| ), CSM goes to this state for post-action.\nYou can use Argument - State to tell which Async Message is called."
      }
      frame "Initialize Core Data" {
        # "#CSM \"Initialize Core Data\"\nThis is used to determine panel behavior on exit"
        # "originally closed?"
        # "exe?"
        # "If panel starts closed or is an EXE, then close it when we exit"
        n125 = property class="VI"() -> ("FP.State"=w327:T2)  [unwired: 2 in, 2 out]
        n126 = property class="App"() -> ("App.Kind"=w333:T3)  [unwired: 2 in, 2 out]
        n127 = control-ref of="Current VI Reference"() -> (w328:refnum<vi>)
        n128 = Equal?(x=w327, y=T2."Closed" ("Front Panel Window:State")) -> (x = y?=w325:bool)
        n129 = Equal?(x=w333, y=T3."Run Time System" ("Application:Kind")) -> (x = y?=w331:bool)
        n130 = Or(x=w325, y=w331) -> (x .or. y?=w329:bool)
        n131 = Bundle By Name(cluster=w330, "Core.Current VI Reference"=w328, "Core.Close Panel on Exit?"=w329) -> (w334:T7)
        n132 = call <vilib>:"Add State(s) to Queue__JKI_lib_State_Machine.vi"("State(s) in (\"\")"=w336) -> ("States Out"=w335:string)  [unwired: 14 in]
      }
      frame "Exit" {
        # "#CSM \"Exit\"\nCase for exiting the loop. No errors that occur here will be handled."
        n133 = call <vilib>:"Add State(s) to Queue__JKI_lib_State_Machine.vi"("State(s) in (\"\")"=w342) -> ("States Out"=w341:string)  [unwired: 14 in]
      }
      frame "---------- Data ----------" {
        # "#CSM \"Category Seperator\"\nDo not put any code in this frame."
        n134 = call <vilib>:"Add State(s) to Queue__JKI_lib_State_Machine.vi"("State(s) in (\"\")"=w347) -> ("States Out"=w346:string)  [unwired: 14 in]
      }
      frame "Data: Initialize" {
        w350 = refnum<queue> refnum  # LoggerWatchDogQueue
        w349 = path ""  # LogFile
        w351 = refnum<vi>[] []  # Toolbar.Advance
        w353 = T8 {"Current VI Reference"=refnum, "Close Panel on Exit?"=FALSE}  # Core
        # "#CSM  do not delete - used by framework"
        # "#CSM Expand Bundle to add new data elements to shift register data."
        # "#CSM Data names and types of shift register data are defined by this bundle."
        # "#CSM \"Data: Initialize\"\nInitialize the shift-register data, here.\n(data names are defined by what you wire into the bundle function)"
        n135 = Bundle("Core"=w353, "Toolbar.Advance"=w351, "LoggerWatchDogQueue"=w350, "LogFile"=w349) -> (w354:T7)  [unwired: 1 in]
        n136 = call <vilib>:"Add State(s) to Queue__JKI_lib_State_Machine.vi"("State(s) in (\"\")"=w356) -> ("States Out"=w355:string)  [unwired: 14 in]
      }
      frame "Data: Initialize References" {
        n137 = control-ref of="Toolbar.Open BD"() -> (w362:refnum<vi>)
        n138 = control-ref of="Toolbar.Open FP"() -> (w361:refnum<vi>)
        n139 = Build Array(w362, w361) -> (w359:refnum<vi>[])
        n140 = Bundle By Name(cluster=w360, "Toolbar.Advance"=w359) -> (w358:T7)
      }
      frame "Data: Cleanup" {
        # "#CSM \"Data: Cleanup\"\nCleanup any data and references, here.\n(this is called automatically, by the Macro: Exit)"
        n141 = Unbundle By Name(w368) -> ("Core.Current VI Reference"=w370:refnum<vi>)
        n142 = Close Reference(reference=w370) -> (error out=w369:errorcluster)  [unwired: 1 in]
        n143 = call <vilib>:"Add State(s) to Queue__JKI_lib_State_Machine.vi"("State(s) in (\"\")"=w372) -> ("States Out"=w371:string)  [unwired: 14 in]
      }
      frame "---------- Events ----------" {
        # "#CSM \"Category Seperator\"\nDo not put any code in this frame."
        n144 = call <vilib>:"Add State(s) to Queue__JKI_lib_State_Machine.vi"("State(s) in (\"\")"=w377) -> ("States Out"=w376:string)  [unwired: 14 in]
      }
      frame "Events: Register" {
        # "#CSM \"Events: Register\"\nRegister user event. New Message Event is registered to break CSM waiting in event structure by default."
        # "#CSM Register New Message Event\nRegister message event to break Waiting in Event structure."
        n145 = call "CSM - Get New State Notifier Event.vi"("Name(\"\" to use uuid) in"=w382) -> ("Error out"=w380:errorcluster, "New State Notifier Event"=w381:refnum<user-event>)  [unwired: 9 in]
        n146 = register-events(error in=w380, w381) -> (reference out=w383:refnum<event-registration>, error out=w379:errorcluster)  [unwired: 1 in]
      }
      frame "Events: Unregister" {
        # "#CSM \"Events: Unregister\"\nUnregister user event."
        n147 = Unregister For Events(event registration refnum=w387) -> (error out=w388:errorcluster)  [unwired: 1 in]
      }
      frame "---------- UI ----------" {
        # "#CSM \"Category Seperator\"\nDo not put any code in this frame."
        n148 = call <vilib>:"Add State(s) to Queue__JKI_lib_State_Machine.vi"("State(s) in (\"\")"=w395) -> ("States Out"=w394:string)  [unwired: 14 in]
      }
      frame "UI: Initialize" {
        # "#CSM \"UI: Initialize\"\nInitialize the User Interface, here.\n(this is called automatically, by the Macro: Init)"
        n149 = call <vilib>:"Add State(s) to Queue__JKI_lib_State_Machine.vi"("State(s) in (\"\")"=w400) -> ("States Out"=w399:string)  [unwired: 14 in]
      }
      frame "UI: Cursor Set" {
        # "Argument"
        # "#CSM \"UI: Cursor Set\"\nSet and Unset Cursor Busy.\n(Usage: \"UI: Cursor Set >> Busy|Idle\")"
        n150 = disable-structure shown="TARGET_TYPE!=Windows" {
          disable-tunnel: [w409 _] -> w404
          disable-tunnel: w403 -> [w408 _]
          frame condition #0 (active) {
            n151 = case shown="\"Idle\", Default" w408 {
              tunnel: [w410 w411] -> w409
              frame "Idle", Default {
                n152 = call <vilib>:"Unset Busy.vi"() -> ("error out"=w410:errorcluster)  [unwired: 11 in]
              }
              frame "Busy" {
                n153 = call <vilib>:"Set Busy.vi"() -> ("error out"=w411:errorcluster)  [unwired: 10 in, 1 out]
              }
            }
          }
          frame condition #1 {
          }
        }
        n154 = call <vilib>:"Add State(s) to Queue__JKI_lib_State_Machine.vi"("State(s) in (\"\")"=w407) -> ("States Out"=w406:string)  [unwired: 14 in]
      }
      frame "UI: Front Panel State" {
        # "Argument"
        # "#CSM \"UI: Front Panel State\"\nSet Front Panel Open or Closed\n(Usage: \"UI: Front Panel State >> Open|Close\")"
        n155 = Unbundle By Name(w416) -> ("Core.Current VI Reference"=w415:refnum<vi>)
        n156 = case shown="\"Minimize\", \"Minimized\"" w414 {
          tunnel: [w426 w439 w450 w462 w474] -> w417
          tunnel: w415 -> [w425 w437 w449 w461 w473]
          frame "Open", "Standard", Default {
            w420 = T2."Standard" ("State")
            n157 = property class="VI"(reference=w425) -> (reference out=w423:refnum<vi>, error out=w424:errorcluster, "FP.State"=w422:T2)  [unwired: 1 in]
            n158 = Not Equal?(x=w422, y=w420) -> (x != y?=w421:bool)
            n159 = case shown="True" w421 {
              tunnel: [w430 w432] -> w426
              tunnel: w424 -> [w429 w432]
              tunnel: w423 -> [w428 _]
              tunnel: w420 -> [w427 _]
              frame True {
                n160 = invoke class="VI" method="FP.Open"(reference=w428, error in=w429, "Activate"=TRUE, "State"=w427) -> (error out=w430:errorcluster)  [unwired: 1 in, 4 out]
              }
              frame False {
              }
            }
          }
          frame "Close", "Closed" {
            n161 = property class="VI"(reference=w437) -> (reference out=w436:refnum<vi>, error out=w438:errorcluster, "FP.State"=w434:T2)  [unwired: 1 in]
            n162 = Not Equal?(x=w434, y=T2."Closed" ("Front Panel Window:State")) -> (x != y?=w433:bool)
            n163 = case shown="True" w433 {
              tunnel: [w440 w443] -> w439
              tunnel: w438 -> [w440 w442]
              tunnel: w436 -> [_ w441]
              frame False {
              }
              frame True {
                n164 = invoke class="VI" method="FP.Close"(reference=w441, error in=w442) -> (error out=w443:errorcluster)  [unwired: 1 in, 2 out]
              }
            }
          }
          frame "Hidden", "Hide" {
            w444 = T2."Hidden" ("State")
            n165 = property class="VI"(reference=w449) -> (reference out=w447:refnum<vi>, error out=w448:errorcluster, "FP.State"=w446:T2)  [unwired: 1 in]
            n166 = Not Equal?(x=w446, y=w444) -> (x != y?=w445:bool)
            n167 = case shown="True" w445 {
              tunnel: [w454 w455] -> w450
              tunnel: w448 -> [w453 w455]
              tunnel: w447 -> [w452 _]
              tunnel: w444 -> [w451 _]
              frame True {
                n168 = invoke class="VI" method="FP.Open"(reference=w452, error in=w453, "State"=w451) -> (error out=w454:errorcluster)  [unwired: 2 in, 4 out]
              }
              frame False {
              }
            }
          }
          frame "Minimize", "Minimized" {
            w456 = T2."Minimized" ("State")
            n169 = property class="VI"(reference=w461) -> (reference out=w459:refnum<vi>, error out=w460:errorcluster, "FP.State"=w458:T2)  [unwired: 1 in]
            n170 = Not Equal?(x=w458, y=w456) -> (x != y?=w457:bool)
            n171 = case shown="False" w457 {
              tunnel: [w466 w467] -> w462
              tunnel: w460 -> [w465 w467]
              tunnel: w459 -> [w464 _]
              tunnel: w456 -> [w463 _]
              frame True {
                n172 = invoke class="VI" method="FP.Open"(reference=w464, error in=w465, "State"=w463) -> (error out=w466:errorcluster)  [unwired: 2 in, 4 out]
              }
              frame False {
              }
            }
          }
          frame "Maximize", "Maximized" {
            w468 = T2."Maximized" ("State")
            n173 = property class="VI"(reference=w473) -> (reference out=w471:refnum<vi>, error out=w472:errorcluster, "FP.State"=w470:T2)  [unwired: 1 in]
            n174 = Not Equal?(x=w470, y=w468) -> (x != y?=w469:bool)
            n175 = case shown="True" w469 {
              tunnel: [w478 w479] -> w474
              tunnel: w472 -> [w477 w479]
              tunnel: w471 -> [w476 _]
              tunnel: w468 -> [w475 _]
              frame True {
                n176 = invoke class="VI" method="FP.Open"(reference=w476, error in=w477, "State"=w475) -> (error out=w478:errorcluster)  [unwired: 2 in, 4 out]
              }
              frame False {
              }
            }
          }
        }
        n177 = call <vilib>:"Add State(s) to Queue__JKI_lib_State_Machine.vi"("State(s) in (\"\")"=w419) -> ("States Out"=w418:string)  [unwired: 14 in]
      }
      frame "UI: Refresh CSM List" {
        n178 = property on="CSM" class="CmbBox"() -> ("Value"=w484:string)  [unwired: 2 in, 2 out]
        n179 = call "CSM - List Modules.vi"() -> ("Error out"=w487:errorcluster, "Module Names"=w482:string[])  [unwired: 10 in]
        n180 = Search 1D Array(1D array=w482, element=w484) -> (index of element=w486:i32)  [unwired: 1 in]
        n181 = Greater Or Equal To 0?(x=w486) -> (x >= 0?=w485:bool)
        n182 = Index Array(array=w482) -> (element=w483:string)  [unwired: 1 in]
        n183 = Select(t=w484, s=w485, f=w483) -> (s? t:f=w481:string)
        n184 = property on="CSM" class="CmbBox"("Strings[]"=w482, "Value"=w481) -> ()  [unwired: 2 in, 2 out]
        n185 = call <vilib>:"Simple Error Handler.vi"("error in (no error)"=w487) -> ()  [unwired: 4 in, 5 out]
      }
      frame "UI: Update Broadcast Registry" {
        n186 = call "CSM - List Mapping Relationships in Broadcast Registry.vi"() -> ("error out"=w493:errorcluster, "Array"=w495:T10)  [unwired: 10 in]
        n187 = for {
          tunnel: w495 -> [w506] mode=indexing
          tunnel: [w499] -> w494 mode=indexing
          n188 = Unbundle(w506) -> ("Status"=w505:string, "Source CSM"=w504:string, "Target CSM"=w503:string, "Target API"=w502:string, "Priority"=w501:T9)
          n189 = Format Into String(w501) -> (resulting string=w500:string)  [unwired: 3 in, 1 out]
          n190 = Build Array(w505, w504, w503, w502, w500) -> (w499:string[])
        }
        "Broadcast Registry" <- w494
      }
      frame "UI: Update Toolbar" {
        w510 = i16 2 ("x")
        n191 = control-ref of="Record.Start"() -> (w511:refnum<vi>)
        n192 = control-ref of="Record.Stop"() -> (w512:refnum<vi>)
        n193 = Unbundle By Name(w508) -> ("Core.Current VI Reference"=w520:refnum<vi>, "LogFile"=w522:path, "LoggerWatchDogQueue"=w513:refnum<queue>)
        n194 = Not A Number/Path/Refnum?(number/path/refnum=w513) -> (NaN/Path/Refnum?=w519:bool)
        n195 = Not(x=w519) -> (.not. x?=w518:bool)
        n196 = Boolean To (0,1)(Boolean=w518) -> (0, 1=w514:i16)
        n197 = Boolean To (0,1)(Boolean=w519) -> (0, 1=w515:i16)
        n198 = Multiply(x=w510, y=w515) -> (x*y=w517:i16)
        n199 = Multiply(x=w510, y=w514) -> (x*y=w516:i16)
        n200 = Empty String/Path?(string/path=w522) -> (empty?=w523:bool)
        n201 = property class="Bool"(reference=w511, "DisabledEnum"=w516) -> ()  [unwired: 1 in, 2 out]
        n202 = property class="Bool"(reference=w512, "DisabledEnum"=w517) -> ()  [unwired: 1 in, 2 out]
        n203 = case shown="True" w523 {
          tunnel: "Running Log Viewer (CSM)" ("Front Panel Window:Title") -> [w531 w532]
          tunnel: [w530 w532] -> w521
          tunnel: w522 -> [w527 _]
          frame False {
            n204 = Path To String(path=w527) -> (string=w528:string)
            n205 = Concatenate Strings(w531, " - " ("string"), w528) -> (w530:string)
          }
          frame True {
          }
        }
        n206 = property class="VI"(reference=w520, "Front Panel.Title"=w521) -> ()  [unwired: 1 in, 2 out]
      }
      frame "UI: Resize Tab Content" {
        w534 = u32 16 ("y")
        w535 = 8 ("Position:Left")
        n207 = control-ref of="Tab"() -> (w536:refnum<vi>)
        n208 = invoke class="TabCtl (strict)" method="FitControlToPane"(reference=w536) -> (reference out=w545:refnum<vi>)  [unwired: 2 in, 2 out]
        n209 = property class="TabCtl (strict)"(reference=w545) -> ("PaneHeight"=w538:u32, "PaneWidth"=w539:u32, "TabHeight"=w543:u32)  [unwired: 1 in, 2 out]
        n210 = control-ref of="Error History"() -> (w537:refnum<vi>)
        n211 = control-ref of="Broadcast Registry"() -> (w540:refnum<vi>)
        n212 = Subtract(x=w538, y=w534) -> (x-y=w541:u32)
        n213 = Subtract(x=w539, y=w534) -> (x-y=w542:u32)
        n214 = Add(x=w535, y=w543) -> (x+y=w544:u32)
        n215 = property class="Str"(reference=w537, "Left"=w535, "Top"=w544, "Height"=w541, "Width"=w542) -> ()  [unwired: 1 in, 2 out]
        n216 = property class="Tbl (strict)"(reference=w540, "Left"=w535, "Top"=w544, "Height"=w541, "Width"=w542) -> ()  [unwired: 1 in, 2 out]
      }
      frame "---------- Macro ----------" {
        # "#CSM \"Category Seperator\"\nDo not put any code in this frame."
        n217 = call <vilib>:"Add State(s) to Queue__JKI_lib_State_Machine.vi"("State(s) in (\"\")"=w554) -> ("States Out"=w553:string)  [unwired: 14 in]
      }
      frame "Macro: Initialize" {
        w557 = "Data: Initialize\nData: Initialize References\nInitialize Core Data\nEvents: Register\nUI: Initialize\nUI: Front Panel State >> Open\nUI: Resize Tab Content\nUI: Refresh CSM List\nUI: Update Broadcast Registry\nUI: Update Toolbar"  # Data: Initialize Data: Initialize References Initialize Core Data Events: Register UI: Initialize UI: Front Panel State >> Open UI: Resize Tab Content UI: Refresh CSM List UI: Update Broadcast Registry UI: Update Toolbar
        # "#CSM \"Macro: Initialize\"\nInitialization Macro (This is called once, when the VI starts)"
        n218 = call <vilib>:"Add State(s) to Queue__JKI_lib_State_Machine.vi"("State(s) in Front (\"\")"=w557, "State(s) in (\"\")"=w560) -> ("States Out"=w559:string)  [unwired: 13 in]
      }
      frame "Macro: Exit" {
        # "#CSM \"Macro: Exit\"\nExit Macro (This is called once, when the VI exits)"
        n219 = Unbundle By Name(w570) -> ("Core.Close Panel on Exit?"=w569:bool)
        n220 = Select(t="UI: Front Panel State >> Close", s=w569, f="") -> (s? t:f=w566:string)
        n221 = call <vilib>:"Add State(s) to Queue__JKI_lib_State_Machine.vi"("State(s) in Front (\"\")"="//Exit Sub-Modules ", "State(s) in (\"\")"=w566, "State(s) at Back (\"\")"="Data: Cleanup\nEvents: Unregister\nExit") -> ("States Out"=w564:string)  [unwired: 12 in]
        n222 = call <vilib>:"Add State(s) to Queue__JKI_lib_State_Machine.vi"("State(s) in Front (\"\")"=w564, "State(s) in (\"\")"=w572) -> ("States Out"=w571:string)  [unwired: 13 in]
      }
      frame "---------- API ----------" {
        # "#CSM \"Category Seperator\"\nDo not put any code in this frame."
      }
      frame "API: API1" {
        # "#CSM >> Source CSM >>\nIf you need to tell who triggered this state , use this string. If it's this case itself, this string is \"\"."
        # "#CSM >> Arguments >>\nDeal with the parameter if any"
        # "#CSM Response\nConnect this to return the response of your API"
        # "#CSM API Example\nCopy/Rename this case for your own API"
      }
      frame "API: API2" {
        # "#CSM API Example\nCopy/Rename this case for your own API"
      }
      frame "---------- Action ----------" {
        # "#CSM \"Category Seperator\"\nDo not put any code in this frame."
        n223 = call <vilib>:"Add State(s) to Queue__JKI_lib_State_Machine.vi"("State(s) in (\"\")"=w590) -> ("States Out"=w589:string)  [unwired: 14 in]
      }
      frame "Action: action1" {
        # "#CSM \"Internal State\"\nThis category is used for holding internal states"
        n224 = call <vilib>:"Add State(s) to Queue__JKI_lib_State_Machine.vi"("State(s) in (\"\")"=w595) -> ("States Out"=w594:string)  [unwired: 14 in]
      }
      frame "Action: action2" {
        # "#CSM \"Internal State\"\nThis category is used for holding internal states"
        n225 = call <vilib>:"Add State(s) to Queue__JKI_lib_State_Machine.vi"("State(s) in (\"\")"=w600) -> ("States Out"=w599:string)  [unwired: 14 in]
      }
    }
  }
  n226 = while "Communicable State Machine(CSM) 2025" {
    shift-right: [w613] -> _
    shift-left: _ -> [w612]
    shift-right: [w616] -> w22
    shift-left: w24 -> [w611]
    shift-right: [w615] -> _
    shift-left: w27 -> [w617]
    shift-right: [w609] -> _
    shift-left: w23 -> [w610]
    tunnel: "Debug-LogViewer" ("Current Module(\"\" to generate a ID)") -> [w608]
    shift-right: [w606] -> _
    shift-left: "" ("String Cache") -> [w607]
    shift-right: [w605] -> _
    shift-left: w18 -> [w602]
    stop <- w614 stop-if-true
    # "Template Copyright © 2018 JKI - http://jki.net/state-machine"
    n227 = call <vilib>:"Parse State Queue__JKI_lib_State_Machine.vi"("State Queue"=w617, "Error In (no error)"=w611) -> ("Remaining States"=w619:string, "Current State"=w620:string, "Arguments"=w618:string)  [unwired: 11 in]
    n228 = Equal To 0?(x=w602) -> (x = 0?=w604:bool)
    n229 = Select(t=-1 ("Timeout"), s=w604, f=w602) -> (s? t:f=w603:i32)
    n230 = case shown="\"\", \"Event Structure\", \"Idle\"" w620 {
      selector: w620 -> [_ _ w845 _ _ _ _ _ _ _ _ _ _ _ _ _ _ _ _ _ _]
      tunnel: w619 -> [w633 w841 w849 w871 w880 w888 w895 w906 w914 w923 w930 w939 w951 w965 w1035 w1041 w1047 w1053 w1061 w1069 w1082]
      tunnel: w618 -> [_ _ _ _ _ _ _ _ _ _ _ _ w946 w959 _ _ _ _ _ _ _]
      tunnel: w612 -> [w631 w838 w847 w864 w877 w886 w892 _ w913 w918 w927 w934 w949 w961 w1034 w1040 w1044 w1052 w1058 w1066 w1079]
      tunnel: [w630 w839 w851 w868 errorcluster {"status"=FALSE, "code"=0, "source"=""} ("error out") w885 w893 w903 w909 w919 w928 w937 w947 w962 w1036 w1042 w1048 w1054 w1059 w1067 w1080] -> w616
      tunnel: w611 -> [w629 w839 w850 w868 w876 w885 w893 w903 w909 w920 w928 w937 w948 w963 w1036 w1042 w1048 w1054 w1059 w1067 w1080]
      tunnel: [w632 w840 w848 w870 w879 w887 w894 w905 w914 w922 w929 w938 w950 w964 w1035 w1041 w1047 w1053 w1060 w1068 w1081] -> w615
      tunnel: [_ _ _ _ _ TRUE _ _ _ _ _ _ _ _ _ _ _ _ _ _ _] -> w614
      tunnel: [w628 w838 w847 w869 w877 w886 w892 w904 w910 w918 w927 w934 w949 w961 w1034 w1040 w1044 w1052 w1058 w1066 w1079] -> w613
      tunnel: w603 -> [w627 w835 w842 w856 w872 w881 w889 w896 w908 w915 w924 w931 w943 w956 w1031 w1037 w1043 w1049 w1055 w1062 w1070]
      tunnel: w610 -> [w626 w837 w844 w858 w874 w883 w891 w901 w912 w917 w926 w936 w945 w958 w1033 w1039 w1046 w1051 w1057 w1064 w1072]
      tunnel: [w625 w837 w844 w858 w874 w883 w891 w901 w912 w917 w926 w936 w945 w958 w1033 w1039 w1046 w1051 w1057 w1064 w1072] -> w609
      tunnel: w608 -> [w624 _ _ _ _ _ _ _ _ _ _ _ _ _ _ _ _ _ _ _ _]
      tunnel: w607 -> [w623 w836 w843 w857 w873 w882 w890 w900 w911 w916 w925 w935 w944 w957 w1032 w1038 w1045 w1050 w1056 w1063 w1071]
      tunnel: [w622 w836 w843 w857 w873 w882 w890 w900 w911 w916 w925 w935 w944 w957 w1032 w1038 w1045 w1050 w1056 w1063 w1071] -> w606
      tunnel: [w621 w835 w842 w856 w872 w881 w889 w896 w908 w915 w924 w931 w943 w956 w1031 w1037 w1043 w1049 w1055 w1062 w1070] -> w605
      frame "", "Event Structure", "Idle" {
        # "executes when the state queue is empty"
        n231 = event shown="[6] <CSM Global Log Event>: User Event" {
          selector: w626 -> [_ _ _ _ _ _ _ _ _ _ _ _ _ _ _ _]
          dyn-events: [_ _ _ _ _ _ _ _ _ _ _ _ _ _ _ _] -> w625
          timeout: w627 -> [_ _ _ _ _ _ _ _ _ _ _ _ _ _ _ _]
          tunnel: w633 -> [w640 w649 w651 w658 w663 w667 w695 w756 w771 w775 w788 w795 w797 w814 w824 w830]
          tunnel: [w639 w648 w650 w658 w663 w667 w694 w756 w771 w775 w788 w795 w796 w813 w825 w831] -> w632
          tunnel: w631 -> [w637 w646 w655 w659 w661 w665 w704 w754 w769 w773 w778 w793 w806 w820 w827 w833]
          tunnel: [w638 w643 w654 w657 w662 w666 w705 w755 w770 w774 w787 w794 w808 w822 w828 w834] -> w630
          tunnel: w629 -> [w638 w647 w654 w657 w662 w666 w705 w755 w770 w774 w787 w794 _ w822 w828 w834]
          tunnel: [w637 w646 w655 w659 w661 w665 w704 w754 w769 w773 w778 w793 w809 w816 w827 w833] -> w628
          tunnel: w624 -> [_ w642 _ _ _ _ _ _ _ _ _ _ _ _ _ _]
          tunnel: w623 -> [w634 w645 w653 w656 w660 w664 w696 w753 w768 w772 w786 _ w811 w821 w826 w832]
          tunnel: [w634 w645 w653 w656 w660 w664 w670 w753 w768 w772 w786 w792 w811 w821 w826 w832] -> w622
          tunnel: [_ -1 ("Timeout") _ _ _ _ w688 _ _ _ _ _ _ _ _ _] -> w621
          event Panel Close? {
            # "Discard the event because we'll close the front panel ourselves in Macro: Exit"
            n232 = event-data() -> ()  [unwired: 1 in, 1 out]
            n233 = call <vilib>:"Add State(s) to Queue__JKI_lib_State_Machine.vi"("State(s) in Front (\"\")"="Macro: Exit", "State(s) in (\"\")"=w640) -> ("States Out"=w639:string)  [unwired: 13 in]
            n234 = event-data("Discard?"=FALSE) -> ()  [unwired: 1 in, 1 out]
          }
          event Timeout {
            n235 = event-data() -> ()  [unwired: 1 in, 1 out]
            n236 = call "CSM - Generate User Global Log.vi"("Place(\"\" to use VI's Name)"=w642, "Error in"=w647, "Log"="No Peroidic Log over 1s.") -> ("error out"=w643:errorcluster)  [unwired: 8 in]
            n237 = call <vilib>:"Add State(s) to Queue__JKI_lib_State_Machine.vi"("State(s) in (\"\")"=w649) -> ("States Out"=w648:string)  [unwired: 14 in]
          }
          event "Search Button": Value Change {
            n238 = event-data() -> ()  [unwired: 1 in, 6 out]
            n239 = call <vilib>:"Add State(s) to Queue__JKI_lib_State_Machine.vi"("State(s) in Front (\"\")"="UI: Refresh CSM List" ("State(s) in Front (\"\")"), "State(s) in (\"\")"=w651) -> ("States Out"=w650:string)  [unwired: 13 in]
          }
          event "Toolbar.Open FP": Value Change {
            n240 = event-data() -> ()  [unwired: 1 in, 6 out]
          }
          event "Toolbar.Open BD": Value Change {
            n241 = event-data() -> ()  [unwired: 1 in, 6 out]
          }
          event "Toolbar.History Length(char)": Value Change {
            n242 = event-data() -> ()  [unwired: 1 in, 6 out]
          }
          event User Event {
            w671 = "%<%H:%M:%S%3u>T" ("Time format string")
            n243 = event-data() -> ("Name(\"\" to use uuid)"=w702:string, "Current State"=w701:string, "Arguments"=w700:string, "Source Message"=w699:T4, "Source Module"=w698:string, "Complete(T)/Start(F)"=w697:bool, "LogType"=w693:T13, "Time Stamp"=w680:timestamp)  [unwired: 1 in]
            n244 = case shown="\"Register\", \"Unregister\"" w693 {
              tunnel: w695 -> [w726 w727 w730 w733]
              tunnel: [w726 w727 w729 w732] -> w694
              frame "State Change", Default {
              }
              frame "User Log" {
              }
              frame "Module Created", "Module Destroyed" {
                n245 = call <vilib>:"Add State(s) to Queue__JKI_lib_State_Machine.vi"("State(s) in Front (\"\")"="UI: Refresh CSM List\nUI: Update Broadcast Registry" ("State(s) in Front (\"\")"), "State(s) in (\"\")"=w730) -> ("States Out"=w729:string)  [unwired: 13 in]
              }
              frame "Register", "Unregister" {
                n246 = call <vilib>:"Add State(s) to Queue__JKI_lib_State_Machine.vi"("State(s) in Front (\"\")"="UI: Update Broadcast Registry" ("State(s) in Front (\"\")"), "State(s) in (\"\")"=w733) -> ("States Out"=w732:string)  [unwired: 13 in]
              }
            }
            n247 = Bundle By Name(cluster=T12 {"Name(\"\" to use uuid)"="", "Current State"="", "Arguments"="", "Source Message"={"‘State"="", "’Arguments"="", "’Error"={"status"=FALSE, "code"=0, "source"=""}}, "Source Module"="", "Complete(T)/Start(F)"=FALSE, "LogType"=enum."State Change", "Time Stamp"=timestamp(0 s since 1904-01-01)} ("Cross CSM Data"), "Name(\"\" to use uuid)"=w702, "Current State"=w701, "Arguments"=w700, "Source Message"=w699, "Source Module"=w698, "Complete(T)/Start(F)"=w697, "LogType"=w693, "Time Stamp"=w680) -> (w691:T12)
            n248 = Not(x="Filter Peroid Logs") -> (.not. x?=w689:bool)
            n249 = call "Periodic Log Filter Check.vi"("Cross CSM Data"=w691, "reset?"=w689, "Settings"=T11 {"threashold(#/s)"=2.0, "Check Peroid(s)"=1.0}) -> ("Cross CSM Data out"=w673:T12, "current time"=w679:timestamp, "additional Info"=w678:string[], "Filtered Status"=w668:string[], "Filtered"=w676:bool)  [unwired: 8 in]
            n250 = case shown="False" w676 {
              tunnel: w673 -> [w713 _]
              tunnel: [w712 _] -> w672
              tunnel: w671 -> [w711 _]
              frame False {
                n251 = call "Global Log To String(Source Time).vi"("format string"=w711, "Log"=w713) -> ("Log String"=w712:string)  [unwired: 8 in]
              }
              frame True {
              }
            }
            n252 = call "PeriodicFilter-Format Result.vi"("Time format string"=w671, "Filtered"=w676, "additional Info"=w678, "current time"=w679, "Cross CSM Data in"=w673) -> ("States"=w677:string)  [unwired: 6 in]
            n253 = case shown="\"Error Log\"" w693 {
              tunnel: "Toolbar.History Length(char)" -> [_ w715]
              tunnel: w672 -> [_ w714]
              frame "User Log", Default {
              }
              frame "Error Log" {
                n254 = local read "Error History"() -> (w719:string)
                n255 = case shown="\"\"" w714 {
                  selector: w714 -> [_ w722]
                  tunnel: "\r" -> [_ w725]
                  tunnel: w719 -> [w721 w724]
                  tunnel: [w721 w723] -> w717
                  frame "" {
                  }
                  frame Default {
                    n256 = Concatenate Strings(w722, w725, w724) -> (w723:string)
                  }
                }
                n257 = String Subset(string=w717, offset (0)=0, length (rest)=w715) -> (substring=→"Error History":string)
              }
            }
            n258 = case shown="\"\"" w677 {
              selector: w677 -> [_ w709]
              tunnel: w696 -> [w706 w710]
              tunnel: [w706 w708] -> w674
              frame "" {
              }
              frame Default {
                n259 = Concatenate Strings(w709, "\r", w710) -> (w708:string)
              }
            }
            n260 = String Subset(string=w674, offset (0)=0, length (rest)="Toolbar.History Length(char)") -> (substring=w670:string)
            n261 = call "PeriodicFilter-Append Filtered Status.vi"("Filtered Status"=w668, "String Cache in"=w670) -> ("String Cache out"=w669:string)  [unwired: 9 in]
            n262 = Empty Array?(array=w668) -> (empty?=w685:bool)
            n263 = Select(t=-1 ("Timeout"), s=w685, f=1000 ("Timeout")) -> (s? t:f=w688:i32)
            n264 = Not(x=w676) -> (.not. x?=w682:bool)
            n265 = call "Check Timeout.vi"("Timeout Expected(ms)"=100, "Force Timeout?"=w682) -> ("Timeout"=w683:bool)  [unwired: 6 in]
            n266 = case shown="True" w683 {
              tunnel: w669 -> [_ _]
              frame False {
              }
              frame True {
              }
            }
          }
          event "State History": Shortcut Menu Activation? {
            n267 = event-data() -> ("CtlRef"=w736:refnum<vi>, "MenuRef"=w735:refnum<k9>, "Coords"=w734:T5)  [unwired: 1 in, 4 out]
            n268 = invoke class="Str" method="ByteOffFromPt"(reference=w736, "Point"=w734) -> (reference out=w752:refnum<vi>, error out=w750:errorcluster, "ByteOffFromPt"=w751:i32)  [unwired: 2 in, 1 out]
            n269 = property class="Str"(reference=w752, error in=w750) -> (error out=w742:errorcluster, "Text.Text"=w748:string)  [unwired: 1 out]
            n270 = String Subset(string=w748, length (rest)=w751) -> (substring=w749:string)  [unwired: 1 in]
            n271 = call "CSM - Break Down Multiple States String.vi"("States"=w748) -> ("Multiple States"=w747:string[])  [unwired: 10 in]
            n272 = call "CSM - Break Down Multiple States String.vi"("States"=w749) -> ("Multiple States"=w746:string[])  [unwired: 10 in]
            n273 = Array Size(array=w746) -> (size(s)=w745:i32)
            n274 = Decrement(x=w745) -> (x-1=w744:i32)
            n275 = Index Array(array=w747, index=w744) -> (element=w743:string)
            n276 = call <vilib>:"Trim Whitespace.vi"("string"=w743) -> ("trimmed string"=w741:string)  [unwired: 1 in]
            n277 = call "_parse Log Line.vi"("string"=w741) -> ("LogType"=w740:string, "State"=w738:string, "CSM"=w739:string)  [unwired: 8 in]
            n278 = case shown="\"State Change\"" w740 {
              tunnel: w735 -> [w766 _]
              tunnel: w741 -> [_ _]
              tunnel: w742 -> [w764 _]
              tunnel: [_ TRUE] -> w737
              tunnel: w739 -> [w762 _]
              tunnel: w738 -> [w761 _]
              frame "State Change" {
                n279 = Format Into String(format string="\"%s@%s\"", w761, w762) -> (resulting string=w757:string)  [unwired: 2 in, 1 out]
                n280 = Concatenate Strings("Go To " ("format string"), w757) -> (w760:string)
                n281 = Concatenate Strings("GO_TO_STATE_" ("item tags"), w757) -> (w758:string)
                n282 = Insert Menu Items(6:w764, 7:w758, 8:w760, 9:w766) -> ()  [unwired: 2 in, 3 out]
              }
              frame Default {
              }
            }
            n283 = event-data("Discard?"=w737) -> ()  [unwired: 1 in, 1 out]
          }
          event "State History": Shortcut Menu Selection (User) {
            n284 = event-data() -> ()  [unwired: 1 in, 8 out]
          }
          event "BackTop": Value Change {
            n285 = event-data() -> ()  [unwired: 1 in, 6 out]
          }
          event Key Down {
            n286 = event-data() -> ("Char"=w776:i16, "PlatMods"=w781:T6)  [unwired: 1 in, 8 out]
            n287 = Unbundle By Name(w781) -> ("Ctrl"=w780:bool)
            n288 = String To Byte Array(string="Qq") -> (unsigned byte array=w783:u8[])
            n289 = Search 1D Array(1D array=w783, element=w776) -> (index of element=w784:i32)  [unwired: 1 in]
            n290 = Unbundle By Name(w778) -> ("Toolbar.Advance"=w777:refnum<vi>[])
            n291 = Greater Or Equal To 0?(x=w784) -> (x >= 0?=w785:bool)
            n292 = And(x=w785, y=w780) -> (x .and. y?=w779:bool)
            n293 = case shown="True" w779 {
              tunnel: w777 -> [_ w789]
              frame False {
              }
              frame True {
                n294 = for {
                  tunnel: w789 -> [w791] mode=indexing
                  n295 = property class="Bool"(reference=w791, "Visible"=TRUE) -> ()  [unwired: 1 in, 2 out]
                }
              }
            }
          }
          event "Clear": Value Change {
            w792 = "" ("String Cache")
            n296 = event-data() -> ()  [unwired: 1 in, 6 out]
            n297 = local write "State History"(w792) -> ()
            n298 = local write "Error History"(w792) -> ()
          }
          event "Record.Start": Value Change {
            n299 = event-data() -> ()  [unwired: 1 in, 1 out]
            n300 = Unbundle By Name(w806) -> ("Core.Current VI Reference"=w805:refnum<vi>)
            n301 = property class="VI"(reference=w805) -> (error out=w804:errorcluster, "OwningApp"=w803:refnum<vi>)  [unwired: 1 in, 1 out]
            n302 = property class="App"(reference=w803, error in=w804) -> (error out=w801:errorcluster, "Project.ActiveProject"=w802:refnum<vi>)  [unwired: 1 out]
            n303 = property class="Project"(reference=w802, error in=w801) -> ("Name"=w800:string)  [unwired: 2 out]
            n304 = String To Path(string=w800) -> (path=w799:path)
            n305 = call "CSM - Start File Logger.vi"("Log File Path"=w799) -> ("Error out"=w808:errorcluster, "LogFile"=w807:path, "WatchDogQueue"=w810:refnum<queue>)  [unwired: 8 in]
            n306 = Bundle By Name(cluster=w806, "LoggerWatchDogQueue"=w810, "LogFile"=w807) -> (w809:T7)
            n307 = call <vilib>:"Add State(s) to Queue__JKI_lib_State_Machine.vi"("State(s) in Front (\"\")"="UI: Update Toolbar" ("State(s) in Front (\"\")"), "State(s) in (\"\")"=w797) -> ("States Out"=w796:string)  [unwired: 13 in]
          }
          event "Record.Stop": Value Change {
            n308 = event-data() -> ()  [unwired: 1 in, 6 out]
            n309 = Unbundle By Name(w820) -> ("LoggerWatchDogQueue"=w819:refnum<queue>)
            n310 = Release Queue(queue=w819, force destroy? (F)=TRUE) -> (error out=w817:errorcluster)  [unwired: 1 in, 2 out]
            n311 = call <vilib>:"Clear Errors.vi"("error in (no error)"=w817) -> ()  [unwired: 5 in, 2 out]
            n312 = Bundle By Name(cluster=w820, "LogFile"=path "") -> (w816:T7)
            n313 = call <vilib>:"Add State(s) to Queue__JKI_lib_State_Machine.vi"("State(s) in Front (\"\")"="UI: Update Toolbar" ("State(s) in Front (\"\")"), "State(s) in (\"\")"=w814) -> ("States Out"=w813:string)  [unwired: 13 in]
          }
          event Pane Size {
            n314 = event-data() -> ()  [unwired: 1 in, 6 out]
            n315 = call <vilib>:"Add State(s) to Queue__JKI_lib_State_Machine.vi"("State(s) in (\"\")"=w824, "State(s) at Back (\"\")"="UI: Resize Tab Content" ("State(s) in Front (\"\")")) -> ("States Out"=w825:string)  [unwired: 13 in]
          }
          event "Tab": Value Change {
            n316 = event-data() -> ()  [unwired: 1 in, 6 out]
            n317 = call <vilib>:"Add State(s) to Queue__JKI_lib_State_Machine.vi"("State(s) in Front (\"\")"="UI: Update Broadcast Registry" ("State(s) in Front (\"\")"), "State(s) in (\"\")"=w830) -> ("States Out"=w831:string)  [unwired: 13 in]
          }
        }
      }
      frame "---------- Core ----------" {
        # "Do not put any code in this frame.\n(it is a separator no-op)"
        n318 = call <vilib>:"Add State(s) to Queue__JKI_lib_State_Machine.vi"("State(s) in (\"\")"=w841) -> ("States Out"=w840:string)  [unwired: 14 in]
      }
      frame Default {
        w854 = 42 items=["No error", "Argument error", "Memory is full", "Out of zone", "End of file", "File already open", "Generic file I/O error", "File not found", "File permission error", "Disk is full", "Duplicate path", "Too many files open", "System feature not enabled", "Resource file not found", "Cannot add resource", "Resource not found", "Image not found", "Image memory error", "Pen does not exist", "Config type invalid", "Config token not found", "Config parse error", "Config memory error", "Bad external code format", "Bad external code offset", "External code not present", "Null window", "Destroy window error", "Null menu", "Print aborted", "Bad print record", "Print driver error", "Windows error during printing", "Memory error during printing", "Print dialog error", "Generic print error", "Invalid device refnum", "Device not found", "Device parameter error", "Device unit error", "Cannot open device", "Device call aborted", "Generic error", "Cancelled by user", "Object ID too low", "Object ID too high", "Object not in heap", "Unknown heap", "Unknown object (invalid DefProc)", "Unknown object (DefProc not in table)", "Message out of range", "Invalid (null) method", "Unknown message", "Manager call not supported", "Bad address", "Network operation in progress", "Network operation timed out", "Connection is busy", "Network attribute not supported", "Network error", "Address in use", "System out of memory", "Connection aborted", "Connection refused", "Not connected", "Already connected", "Connection closed", "Initialization error (interapplication manager)", "Bad occurrence", "Wait on unbound occurrence handler", "Occurrence queue overflow", "Datalog type conflict", "Unused", "Unrecognized type (interapplication manager)", "Memory corrupt", "Failed to make temporary DLL", "Old CIN version", "Drag socket not found", "Failed to load drop-object", "Failed to register OLE object", "Failed to release OLE object", "Format specifier type mismatch", "Unknown format specifier", "Too few format specifiers", "Too many format specifiers", "Scan failed", "Newer CIN version", "Error converting to variant", "Runtime menu error", "Password tampered", "Variant attribute not found", "Incompatible variant data type", "Event data is not available", "Event Store is not present", "Occurrence is not found", "Event Queue is not created", "Event info is not available", "Refnum passed is NULL", "Error retrieving Class GUID", "Error retrieving CoClass GUID", "Error retrieving TypeLib GUID.", "Bad built application magic bytes.", "Specific driver is different from the specific driver associated with the Logical Name.", "There is no session opened to the class driver.", "Max Error", "MAX - Error with config objects", "MAX - Error loading configuration", "MAX - Group not supported"]
        # "Current State"
        # "Do not delete, rename, or modify this frame.\n(this is used to capture unhandled states and typos)"
        # "Handle mistyped state name (developer tool)"
        n319 = Format Into String(format string="Software Exception: Unhandled State \"%s\"." ("message"), error in=w850, w845) -> (resulting string=w853:string, error out=w852:errorcluster)  [unwired: 1 in]
        n320 = call <vilib>:"Error Cluster From Error Code.vi"("show call chain? (False)"=TRUE, "error in (no error)"=w852, "error message (\"\")"=w853, "error code (0)"=w854) -> ("error out"=w851:errorcluster)  [unwired: 5 in]
        n321 = call <vilib>:"Add State(s) to Queue__JKI_lib_State_Machine.vi"("State(s) in (\"\")"=w849) -> ("States Out"=w848:string)  [unwired: 14 in]
      }
      frame "Initialize Core Data" {
        # "Do not delete, rename, or modify this frame.\n(this is used to determine panel behavior on exit)"
        # "originally closed?"
        # "exe?"
        # "If panel starts closed or is an EXE, then close it when we exit"
        n322 = property class="VI"() -> ("FP.State"=w861:T2)  [unwired: 2 in, 2 out]
        n323 = property class="App"() -> ("App.Kind"=w867:T3)  [unwired: 2 in, 2 out]
        n324 = control-ref of="Current VI Reference"() -> (w862:refnum<vi>)
        n325 = Equal?(x=w861, y=T2."Closed" ("Front Panel Window:State")) -> (x = y?=w859:bool)
        n326 = Equal?(x=w867, y=T3."Run Time System" ("Application:Kind")) -> (x = y?=w865:bool)
        n327 = Or(x=w859, y=w865) -> (x .or. y?=w863:bool)
        n328 = Bundle By Name(cluster=w864, "Core.Current VI Reference"=w862, "Core.Close Panel on Exit?"=w863) -> (w869:T7)
        n329 = call <vilib>:"Add State(s) to Queue__JKI_lib_State_Machine.vi"("State(s) in (\"\")"=w871) -> ("States Out"=w870:string)  [unwired: 14 in]
      }
      frame "Error Handler" {
        # "Unhandled Error -- Display it"
        # "Handle any errors here.\nYou can also output any states to clean-up after errors occur"
        # "Clear error"
        n330 = call <vilib>:"General Error Handler.vi"("error in (no error)"=w876) -> ()  [unwired: 10 in, 5 out]
        n331 = call <vilib>:"Add State(s) to Queue__JKI_lib_State_Machine.vi"("State(s) in Front (\"\")"="/* Post Error States", "State(s) in (\"\")"=w880) -> ("States Out"=w879:string)  [unwired: 13 in]
      }
      frame "Exit" {
        # "Do not put any code in this frame.\n(No errors that occur here will be handled.)"
        n332 = call <vilib>:"Add State(s) to Queue__JKI_lib_State_Machine.vi"("State(s) in (\"\")"=w888) -> ("States Out"=w887:string)  [unwired: 14 in]
      }
      frame "---------- Data ----------" {
        # "Do not put any code in this frame.\n(It is a separator no-op. You can make a copy of this frame to create a new Data frame)"
        n333 = call <vilib>:"Add State(s) to Queue__JKI_lib_State_Machine.vi"("State(s) in (\"\")"=w895) -> ("States Out"=w894:string)  [unwired: 14 in]
      }
      frame "Data: Initialize" {
        w897 = refnum<queue> refnum  # LoggerWatchDogQueue
        w898 = path ""  # LogFile
        w899 = refnum<vi>[] []  # Toolbar.Advance
        w902 = T8 {"Current VI Reference"=refnum, "Close Panel on Exit?"=FALSE}  # Core
        # "Data names and types of shift register data are defined by this bundle."
        # "Initialize the shift-register data, here.\n(data names are defined by what you wire into the bundle function)"
        n334 = Bundle("Core"=w902, "Toolbar.Advance"=w899, "LoggerWatchDogQueue"=w897, "LogFile"=w898) -> (w904:T7)  [unwired: 1 in]
        n335 = call <vilib>:"Add State(s) to Queue__JKI_lib_State_Machine.vi"("State(s) in (\"\")"=w906) -> ("States Out"=w905:string)  [unwired: 14 in]
      }
      frame "Data: Initialize References" {
        n336 = Bundle By Name(cluster=w913, "Toolbar.Advance"=refnum<vi>[] []) -> (w910:T7)
      }
      frame "Data: Cleanup" {
        # "Cleanup any data and references, here.\n(this is called automatically, by the Macro: Exit)"
        n337 = Unbundle By Name(w918) -> ("Core.Current VI Reference"=w921:refnum<vi>)
        n338 = Close Reference(reference=w921, error in (no error)=w920) -> (error out=w919:errorcluster)
        n339 = call <vilib>:"Add State(s) to Queue__JKI_lib_State_Machine.vi"("State(s) in (\"\")"=w923) -> ("States Out"=w922:string)  [unwired: 14 in]
      }
      frame "---------- UI ----------" {
        # "Do not put any code in this frame.\n(It is a separator no-op. You can make a copy of this frame to create a new UI frame)"
        n340 = call <vilib>:"Add State(s) to Queue__JKI_lib_State_Machine.vi"("State(s) in (\"\")"=w930) -> ("States Out"=w929:string)  [unwired: 14 in]
      }
      frame "UI: Initialize" {
        # "Initialize the User Interface, here.\n(this is called automatically, by the Macro: Init)"
        n341 = Unbundle By Name(w934) -> ("Toolbar.Advance"=w933:refnum<vi>[])
        n342 = disable-structure shown="Disabled" {
          disable-tunnel: w933 -> [w940 _]
          frame Disabled {
            n343 = for {
              tunnel: w940 -> [w942] mode=indexing
              n344 = property class="Bool"(reference=w942, "Visible"=FALSE) -> ()  [unwired: 1 in, 2 out]
            }
          }
          frame Enabled {
          }
        }
        n345 = local write "Filter Peroid Logs"(TRUE ("Filter Peroid Logs")) -> ()
        n346 = call <vilib>:"Add State(s) to Queue__JKI_lib_State_Machine.vi"("State(s) in (\"\")"=w939) -> ("States Out"=w938:string)  [unwired: 14 in]
      }
      frame "UI: Cursor Set" {
        # "Argument"
        # "Set and Unset Cursor Busy.\n(Usage: \"UI: Cursor Set >> Busy|Idle\")"
        n347 = case shown="\"Idle\", Default" w946 {
          tunnel: w948 -> [w953 w955]
          tunnel: [w952 w954] -> w947
          frame "Idle", Default {
            n348 = call <vilib>:"Unset Busy.vi"("error in (no error)"=w953) -> ("error out"=w952:errorcluster)  [unwired: 10 in]
          }
          frame "Busy" {
            n349 = call <vilib>:"Set Busy.vi"("error in (no error)"=w955) -> ("error out"=w954:errorcluster)  [unwired: 9 in, 1 out]
          }
        }
        n350 = call <vilib>:"Add State(s) to Queue__JKI_lib_State_Machine.vi"("State(s) in (\"\")"=w951) -> ("States Out"=w950:string)  [unwired: 14 in]
      }
      frame "UI: Front Panel State" {
        # "Argument"
        # "Set Front Panel Open or Closed\n(Usage: \"UI: Front Panel State >> Open|Close\")"
        n351 = Unbundle By Name(w961) -> ("Core.Current VI Reference"=w960:refnum<vi>)
        n352 = case shown="\"Minimize\", \"Minimized\"" w959 {
          tunnel: w963 -> [w971 w986 w997 w1010 w1023]
          tunnel: [w973 w987 w999 w1012 w1025] -> w962
          tunnel: w960 -> [w972 w984 w998 w1011 w1024]
          frame "Open", "Standard", Default {
            w966 = T2."Standard" ("State")
            n353 = property class="VI"(reference=w972, error in=w971) -> (reference out=w969:refnum<vi>, error out=w970:errorcluster, "FP.State"=w968:T2)
            n354 = Not Equal?(x=w968, y=w966) -> (x != y?=w967:bool)
            n355 = case shown="True" w967 {
              tunnel: [w977 w979] -> w973
              tunnel: w970 -> [w976 w979]
              tunnel: w969 -> [w975 _]
              tunnel: w966 -> [w974 _]
              frame True {
                n356 = invoke class="VI" method="FP.Open"(reference=w975, error in=w976, "Activate"=TRUE, "State"=w974) -> (error out=w977:errorcluster)  [unwired: 1 in, 4 out]
              }
              frame False {
              }
            }
          }
          frame "Close", "Closed" {
            n357 = property class="VI"(reference=w984, error in=w986) -> (reference out=w983:refnum<vi>, error out=w985:errorcluster, "FP.State"=w981:T2)
            n358 = Not Equal?(x=w981, y=T2."Closed" ("Front Panel Window:State")) -> (x != y?=w980:bool)
            n359 = case shown="True" w980 {
              tunnel: [w988 w991] -> w987
              tunnel: w985 -> [w988 w990]
              tunnel: w983 -> [_ w989]
              frame False {
              }
              frame True {
                n360 = invoke class="VI" method="FP.Close"(reference=w989, error in=w990) -> (error out=w991:errorcluster)  [unwired: 1 in, 2 out]
              }
            }
          }
          frame "Hidden", "Hide" {
            w992 = T2."Hidden" ("State")
            n361 = property class="VI"(reference=w998, error in=w997) -> (reference out=w995:refnum<vi>, error out=w996:errorcluster, "FP.State"=w994:T2)
            n362 = Not Equal?(x=w994, y=w992) -> (x != y?=w993:bool)
            n363 = case shown="True" w993 {
              tunnel: [w1003 w1004] -> w999
              tunnel: w996 -> [w1002 w1004]
              tunnel: w995 -> [w1001 _]
              tunnel: w992 -> [w1000 _]
              frame True {
                n364 = invoke class="VI" method="FP.Open"(reference=w1001, error in=w1002, "State"=w1000) -> (error out=w1003:errorcluster)  [unwired: 2 in, 4 out]
              }
              frame False {
              }
            }
          }
          frame "Minimize", "Minimized" {
            w1005 = T2."Minimized" ("State")
            n365 = property class="VI"(reference=w1011, error in=w1010) -> (reference out=w1008:refnum<vi>, error out=w1009:errorcluster, "FP.State"=w1007:T2)
            n366 = Not Equal?(x=w1007, y=w1005) -> (x != y?=w1006:bool)
            n367 = case shown="True" w1006 {
              tunnel: [w1016 w1017] -> w1012
              tunnel: w1009 -> [w1015 w1017]
              tunnel: w1008 -> [w1014 _]
              tunnel: w1005 -> [w1013 _]
              frame True {
                n368 = invoke class="VI" method="FP.Open"(reference=w1014, error in=w1015, "State"=w1013) -> (error out=w1016:errorcluster)  [unwired: 2 in, 4 out]
              }
              frame False {
              }
            }
          }
          frame "Maximize", "Maximized" {
            w1018 = T2."Maximized" ("State")
            n369 = property class="VI"(reference=w1024, error in=w1023) -> (reference out=w1021:refnum<vi>, error out=w1022:errorcluster, "FP.State"=w1020:T2)
            n370 = Not Equal?(x=w1020, y=w1018) -> (x != y?=w1019:bool)
            n371 = case shown="True" w1019 {
              tunnel: [w1029 w1030] -> w1025
              tunnel: w1022 -> [w1028 w1030]
              tunnel: w1021 -> [w1027 _]
              tunnel: w1018 -> [w1026 _]
              frame True {
                n372 = invoke class="VI" method="FP.Open"(reference=w1027, error in=w1028, "State"=w1026) -> (error out=w1029:errorcluster)  [unwired: 2 in, 4 out]
              }
              frame False {
              }
            }
          }
        }
        n373 = call <vilib>:"Add State(s) to Queue__JKI_lib_State_Machine.vi"("State(s) in (\"\")"=w965) -> ("States Out"=w964:string)  [unwired: 14 in]
      }
      frame "UI: Refresh CSM List" {
      }
      frame "UI: Update Broadcast Registry" {
      }
      frame "UI: Update Toolbar" {
      }
      frame "UI: Resize Tab Content" {
      }
      frame "---------- Macro ----------" {
        # "Do not put any code in this frame.\n(It is a separator no-op. You can make a copy of this frame to create a new Macro frame)"
        n374 = call <vilib>:"Add State(s) to Queue__JKI_lib_State_Machine.vi"("State(s) in (\"\")"=w1061) -> ("States Out"=w1060:string)  [unwired: 14 in]
      }
      frame "Macro: Initialize" {
        w1065 = "Data: Initialize\nData: Initialize References\nInitialize Core Data\nUI: Initialize\nUI: Front Panel State >> Open\nUI: Resize Tab Content\nUI: Refresh CSM List\nUI: Update Broadcast Registry\nUI: Update Toolbar"  # Data: Initialize Data: Initialize References Initialize Core Data UI: Initialize UI: Front Panel State >> Open UI: Resize Tab Content UI: Refresh CSM List UI: Update Broadcast Registry UI: Update Toolbar
        # "Initialization Macro\n(This is called once, when the VI starts)"
        n375 = call <vilib>:"Add State(s) to Queue__JKI_lib_State_Machine.vi"("State(s) in Front (\"\")"=w1065, "State(s) in (\"\")"=w1069) -> ("States Out"=w1068:string)  [unwired: 13 in]
      }
      frame "Macro: Exit" {
        # "Exit Macro\n(This is called once, when the VI exits)"
        n376 = Unbundle By Name(w1079) -> ("Core.Close Panel on Exit?"=w1078:bool)
        n377 = Select(t="UI: Front Panel State >> Close", s=w1078, f="") -> (s? t:f=w1075:string)
        n378 = call <vilib>:"Add State(s) to Queue__JKI_lib_State_Machine.vi"("State(s) in (\"\")"=w1075, "State(s) at Back (\"\")"="Data: Cleanup\nExit") -> ("States Out"=w1073:string)  [unwired: 13 in]
        n379 = call <vilib>:"Add State(s) to Queue__JKI_lib_State_Machine.vi"("State(s) in Front (\"\")"=w1073, "State(s) in (\"\")"=w1082) -> ("States Out"=w1081:string)  [unwired: 13 in]
      }
    }
  }
  n380 = while {
    shift-right: [w1118] -> w5
    shift-left: w11 -> [w1115]
    shift-right: [w1108] -> w4
    shift-left: w12 -> [w1119]
    shift-right: [w1103] -> w3
    shift-left: w8 -> [w1103]
    tunnel: w7 -> [w1083]
    stop <- w1105 stop-if-true
    n381 = Get Queue Status(queue=w1119, error in (no error)=w1115) -> (queue out=w1117:refnum<queue>, error out=w1116:errorcluster, # elements in queue=w1089:i32)  [unwired: 1 in, 5 out]
    "LogInQ" <- w1089
    n382 = call "Auto Processing Level.vi"("#Left In Q"=w1089) -> ("Level"=w1097:T1)  [unwired: 8 in, 2 out]
    n383 = feedback #1(Periodic_String_Filter_Level."normal" ("Level")) -> (w1100:T1)
    n384 = feedback-in #1(w1097) -> ()
    n385 = Not Equal?(x=w1097, y=w1100) -> (x != y?=w1098:bool)
    n386 = case shown="True" w1098 {
      tunnel: w1097 -> [_ w1137]
      frame False {
      }
      frame True {
        n387 = local write "Level"(w1137) -> ()
      }
    }
    n388 = Dequeue Element(queue=w1117, timeout in ms (-1)=100, error in (no error)=w1116) -> (queue out=w1108:refnum<queue>, element=w1114:T12, timed out?=w1101:bool, error out=w1118:errorcluster)
    n389 = Not(x=w1101) -> (.not. x?=w1102:bool)
    n390 = call "Occurrence Speed Counter.vi"("period(0.1s)"=1.0, "Occured?(T)"=w1102) -> ("Speed(#/s)"=w1088:dbl)  [unwired: 7 in, 2 out]
    "Handling Speed(#/s)" <- w1088
    n391 = Bundle("Threashold(#/s)"="Threashold(#/s)", "Check Peroid(s)"="Check Peroid(s)") -> (w1085:T14)  [unwired: 1 in]
    n392 = Equal To 0?(x=w1088) -> (x = 0?=w1095:bool)
    n393 = Unbundle By Name(w1085) -> ("Check Peroid(s)"=w1090:dbl)
    n394 = Add(x=w1090, y=w1090) -> (x+y=w1091:dbl)
    n395 = call "Debounced Signal.vi"("Debounce Period(5s)"=w1091, "Signal"=w1095) -> ("Since Last Change(s)"=w1092:dbl, "signal(safe)"=w1094:bool)  [unwired: 8 in]
    n396 = call "Rising Edge.vi"("signal"=w1094) -> ("rising edge"=w1093:bool)
    n397 = case shown="True" w1093 {
      tunnel: w1092 -> [_ w1121]
      frame False {
      }
      frame True {
        n398 = Format Into String(format string="No Log for %.0fs", w1121) -> (resulting string=w1122:string)  [unwired: 2 in, 1 out]
        n399 = call "CSM - Generate User Global Log.vi"("Place(\"\" to use VI's Name)"="CSM Debug Console", "Log"=w1122) -> ()  [unwired: 9 in, 1 out]
      }
    }
    n400 = feedback #2("" ("String Cache")) -> (w1110:string)
    n401 = case shown="False" w1101 {
      tunnel: w1114 -> [w1130 _]
      tunnel: [w1132 w1135] -> w1111
      tunnel: w1110 -> [_ w1135]
      tunnel: w1103 -> [w1129 _]
      tunnel: w1085 -> [w1127 _]
      frame False {
        n402 = Unbundle By Name(w1130) -> ("LogType"=w1131:T13)
        n403 = case shown="\"Module Created\", \"Module Destroyed\"" w1131 {
          tunnel: w1129 -> [_ w1134]
          frame "User Log", Default {
          }
          frame "Module Created", "Module Destroyed" {
            n404 = Generate User Event(user event=w1134, event data cluster="UI: Refresh CSM List" ("State(s) in Front (\"\")")) -> ()  [unwired: 2 in, 2 out]
          }
        }
        n405 = Not(x="Periodic") -> (.not. x?=w1128:bool)
        n406 = call "Global Log History Cacher.vi"("Cross CSM Data"=w1130, "reset?"=w1128, "with Periodic Info(T)"="Periodic Info", "Settings"=w1127, "Level(Normal)"="Level") -> ("String Cache"=w1132:string)  [unwired: 10 in]
      }
      frame True {
      }
    }
    n407 = feedback-in #2(w1111) -> ()
    n408 = call "CSM - Module Turns Invalid.vi"("CSM Name"=w1083) -> ("Turn Invalid(Exit)?"=w1084:bool)  [unwired: 2 in]
    n409 = Compound Arithmetic op=OR(w1118, w1084) -> (w1106:bool)
    n410 = call "Exit With Empty Queue Check.vi"("queue"=w1108, "timeout(5s)"=1.0, "Stop"=w1106) -> ("exit"=w1105:bool)  [unwired: 7 in, 1 out]
    n411 = call "Check Timeout.vi"() -> ("Timeout"=w1112:bool)  [unwired: 8 in]
    n412 = Or(x=w1105, y=w1112) -> (x .or. y?=w1107:bool)
    n413 = case shown="True" w1107 {
      tunnel: w1111 -> [_ w1136]
      frame False {
      }
      frame True {
        "State History" <- w1136
      }
    }
  }
  n414 = call "CSM - Destroy Global Log Event.vi"("Error in"=w22, "CSM Global Log Event"=w28) -> ("Error out"=w21:errorcluster)  [unwired: 9 in]
  n415 = invoke class="VI" method="FP.Close"(error in=w21) -> (error out=w30:errorcluster)  [unwired: 2 in, 2 out]
  n416 = call "CSM - Destroy Global Log Queue.vi"("Error in"=w5, "CreatedQueue"=w4) -> ("Error out"=w6:errorcluster)  [unwired: 9 in]
  n417 = invoke class="VI" method="FP.Close"(error in=w13) -> (error out=w14:errorcluster)  [unwired: 2 in, 2 out]
  n418 = call <vilib>:"Clear Errors.vi"("error in (no error)"=w30) -> ()  [unwired: 5 in, 2 out]
  n419 = Destroy User Event(user event=w3, error in=w6) -> (error out=w1:errorcluster)
  n420 = Merge Errors(w14, w1) -> (w2:errorcluster)
  n421 = call <vilib>:"Clear Errors.vi"("error in (no error)"=w2) -> ()  [unwired: 5 in, 2 out]
